vi "Update Main _ Avg Sweeps.vi"() -> ()   [LabVIEW 2022 SP3]
uses:
  Logo.ctl
  C:/Users/Public/OneDrive/Desktop/PMT program/SampleCodeLabView/Kinesis_with_LabVIEW_Examples_LV12 - v3/Thorlabs.MotionControl.Controls.dll
  Kinesis_with_LabVIEW_Examples_LV12 - v3/Thorlabs.MotionControl.Controls.dll
  <vilib>/Utility/file.llb/Write Delimited Spreadsheet (string).vi
  <vilib>/Utility/file.llb/Write Delimited Spreadsheet (I64).vi
  <vilib>/Utility/file.llb/Write Delimited Spreadsheet (DBL).vi
  C:/Users/Public/OneDrive/Desktop/PMT program/SampleCodeLabView/Kinesis_with_LabVIEW_Examples_LV12 - v3/ThorLabs.MotionControl.KCube.DCServoCLI.dll
  Kinesis_with_LabVIEW_Examples_LV12 - v3/ThorLabs.MotionControl.KCube.DCServoCLI.dll
  <vilib>/Analysis/NI_AALBase.lvlib
panel:
  out "RSD":i32=5 caption="Repeat Sweep Data"
  in  "Tab Control":enum32{"Page 1", "Page 2", "Page 3"}(tab)
  out "Sweep Graph":u32[](graph)
  out "Cycled Mean Graph":u32[](graph)
  out "Multiplot":waveform(dbl)[](graph)
  in  "RS":i32=5 caption="Repeat Cycle"
  out "SIND":i32 caption="Total No. of Sweep Iterations"
  out "SIN":i32 caption="Current Sweep Iteration"
  out "ESD":i32=1 caption="Steps\nAdded/Removed"
  in  "ES":i32=1 caption="Add /Remove \nSteps"
  out "SM":i32 caption="Sweep\nMean"
  out "SN":i32 caption="Current  Read Step"
  out "SND":i32 caption="Total No. of Read Steps"
  in  "Auto-Sweep":bool
  in  "P8":bool
  out "PC":i32 caption="Current \nPosition"
  out "WTD":i32=2500 caption="Wait Time (ms)\nRead Data"
  out "EPD":i32=180 caption="End Position\nRead Data"
  out "SPD":i32 caption="Start Position\nRead Data"
  out "SSD":i32=10 caption="Step Size\nRead Data"
  in  "SP":i32 caption="Start Position (degrees)\n Set Data"
  in  "WT":i32=2500 caption="Wait Time (ms)\n Set Data"
  in  "EP":i32=180 caption="End Position (degrees)\n Set Data"
  in  "P7":bool
  in  "SS":i32=10 caption="Step Size (degrees)\nSet Data"
  in  "Motor Controller\nSerialNumber":string="27260805"
  in  "KCubeDCServoControl":refnum<k24>(container)
  in  "Export":bool
  out "DB":u32[](array[numeric])
  out "OVL":bool caption="LED ON : Over Rang Data"
  out "OLD":i32
  out "GN":i32 caption="Gate Number"
  in  "Correction":bool=TRUE
  in  "Logo":T1
  out "Graph":u32[](graph)
  in  "Stop":bool
  in  "Start":bool
  in  "P6":bool
  out "RND":i32=50 caption="Read Number\nRead Data"
  in  "P5":bool
  in  "RN":i32=50 caption="Read Number\nSet Data"
  out "PowerD":i32 caption="Power\nRead Data"
  out "ITD":i32=40 caption="Internal Time\nRead Data"
  in  "P4":bool
  in  "P3":bool
  in  "IT":i32=40 caption="Internal Time\nSet Data"
  in  "P2":bool
  out "Handle Number":i32
  in  "P1":bool caption="Switch\nPower OFF/Power ON"
  in  "EXIT":bool
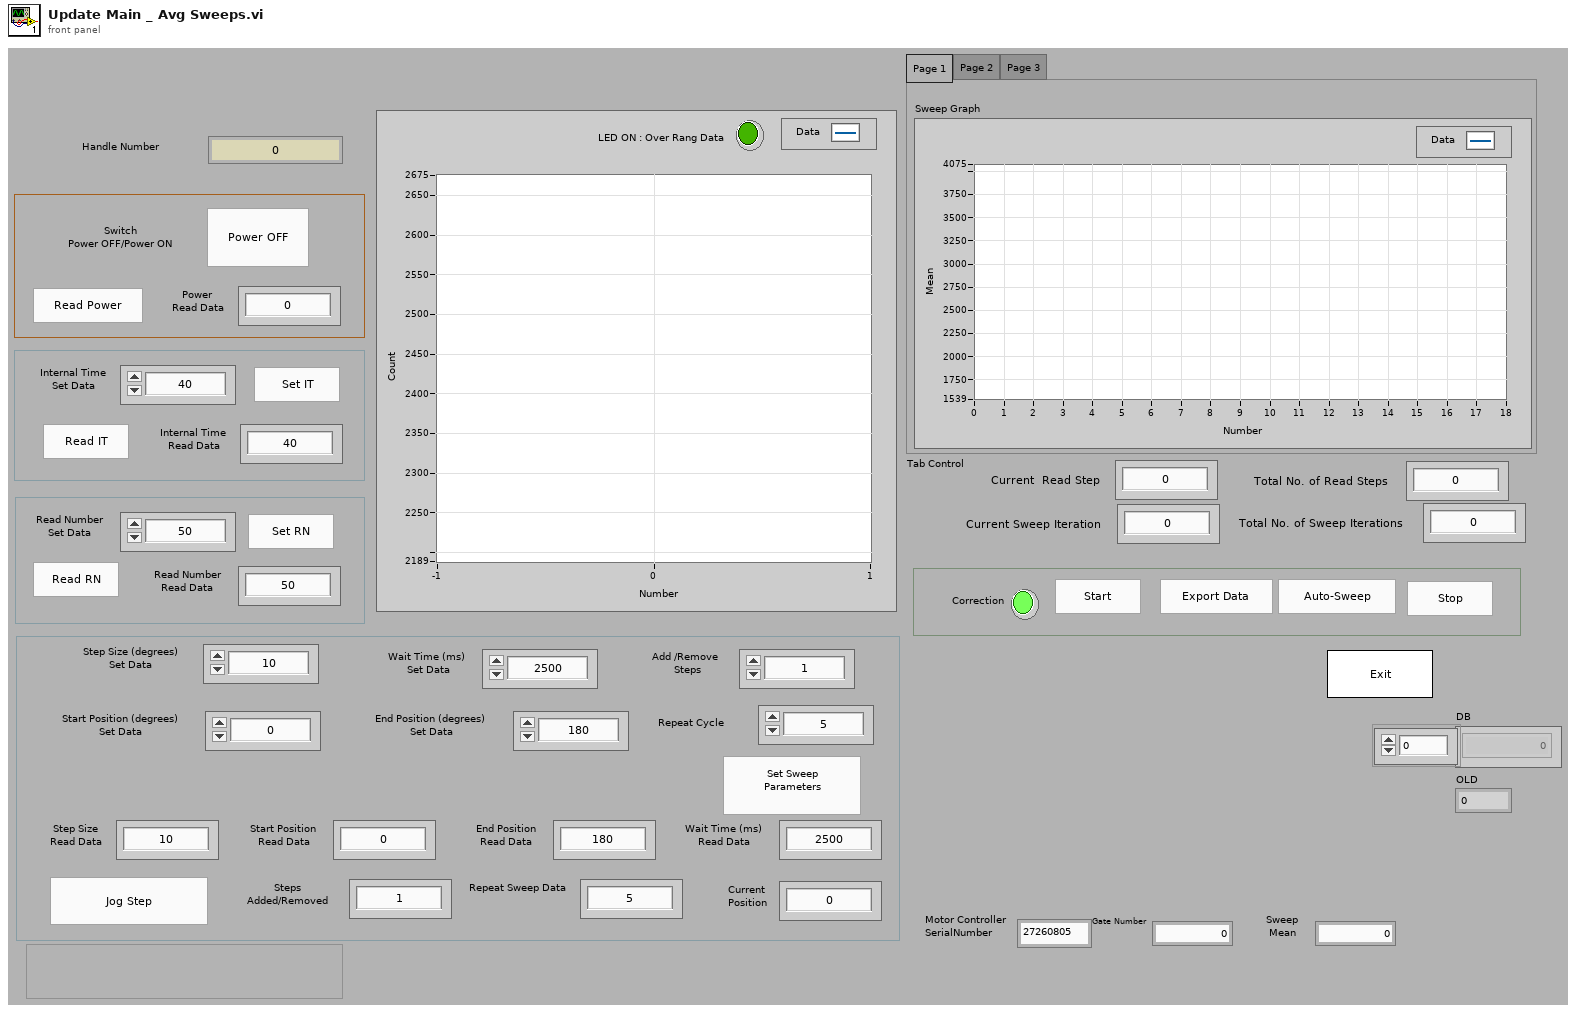
[diagram p1: front panel]
types:
  T1 = typedef "Logo.ctl" = bool
  T2 = enum8{"Enabled", "Disabled", "Disabled and Grayed Out"}
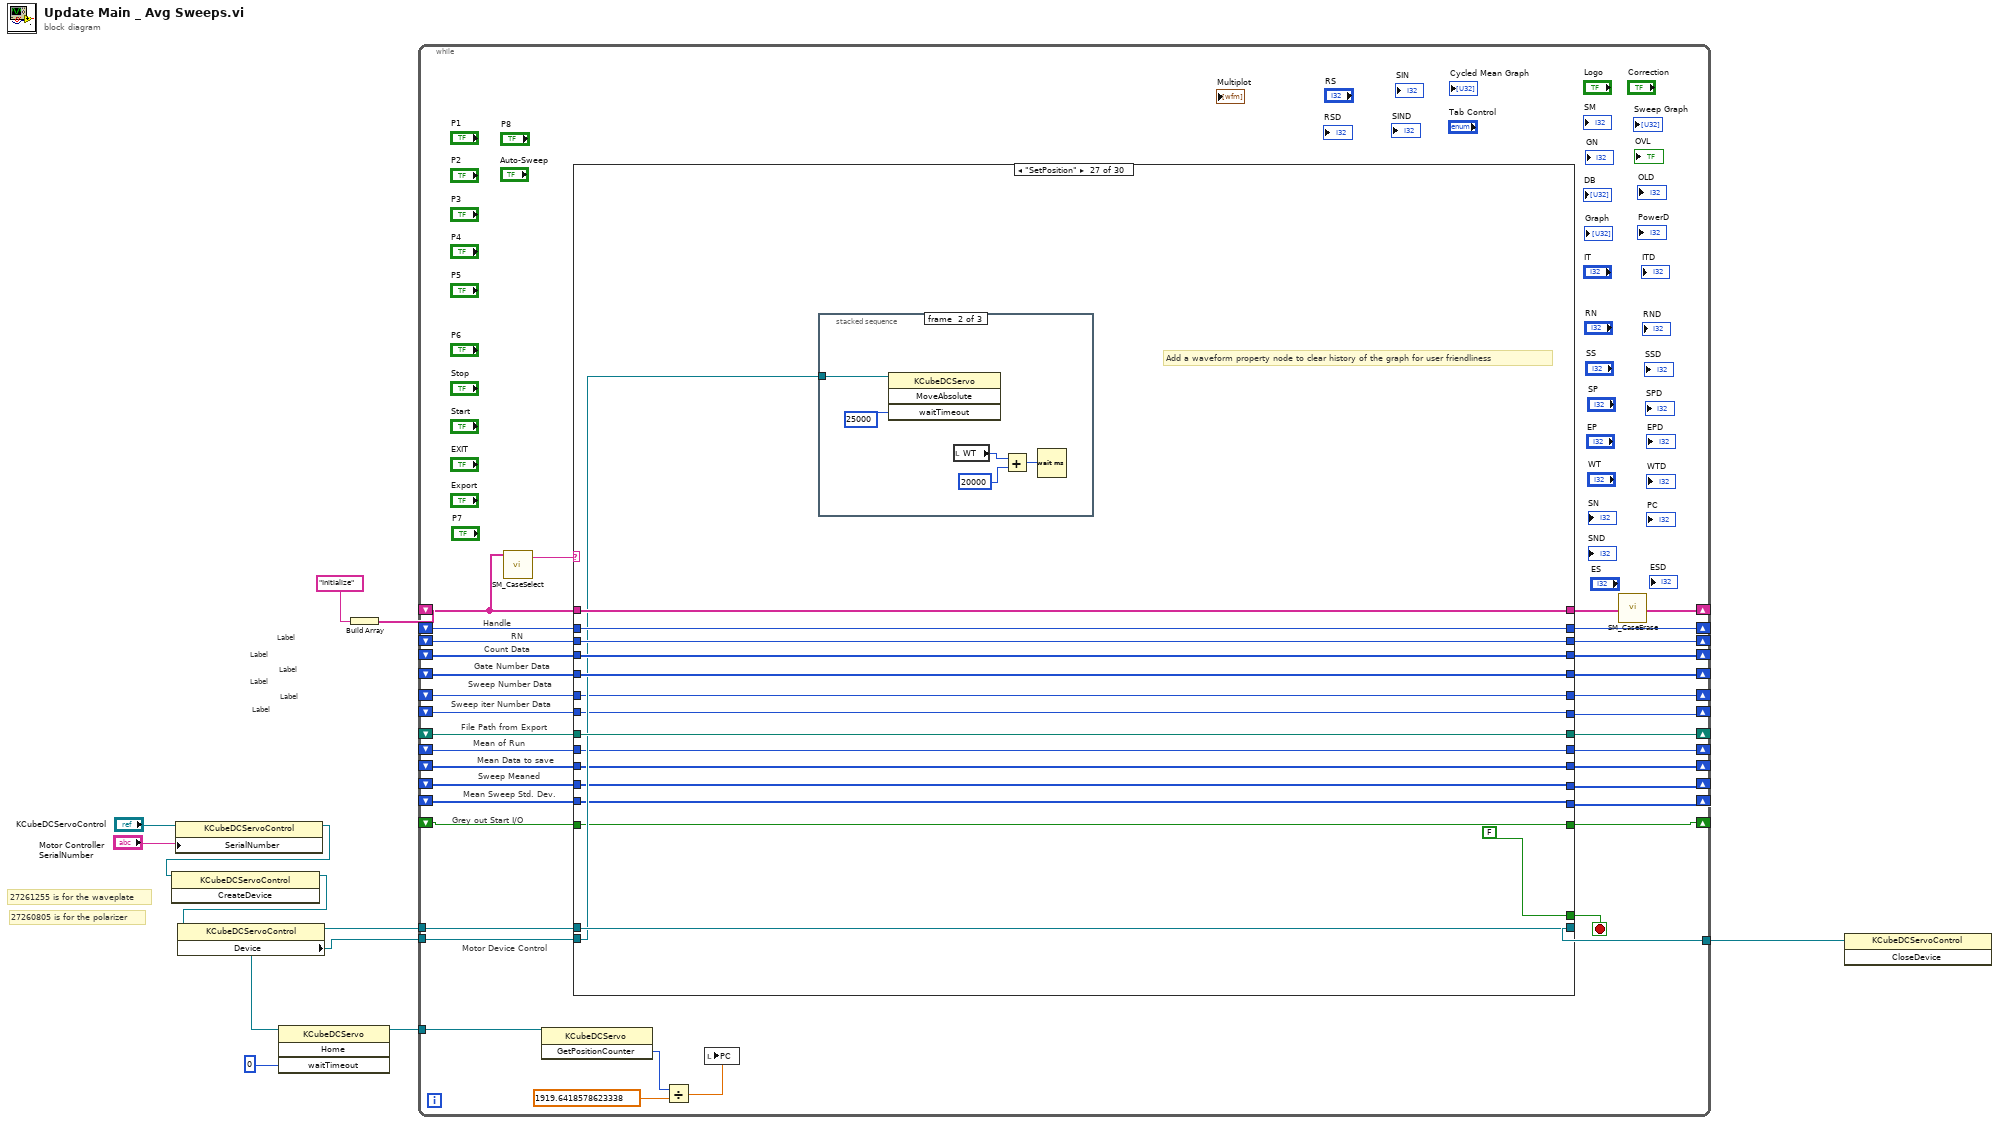
[diagram p0: block diagram]
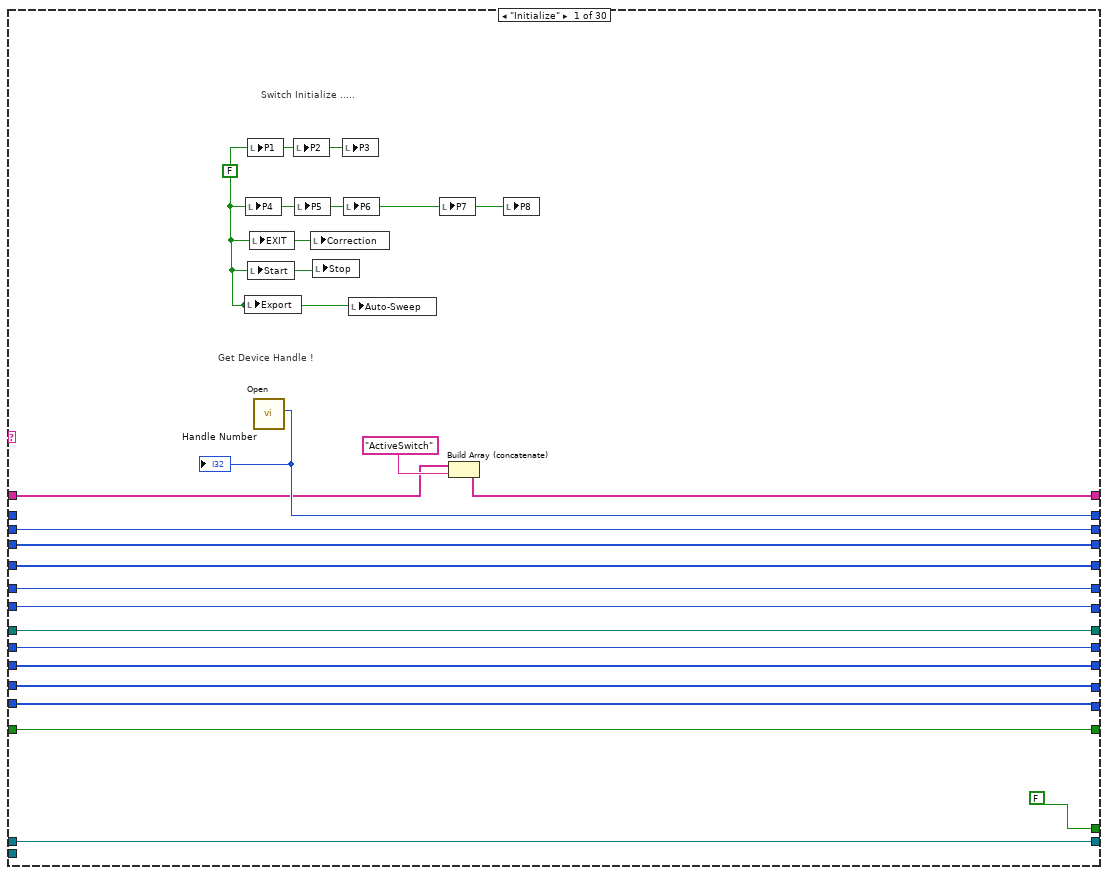
[diagram p2: hidden frame]
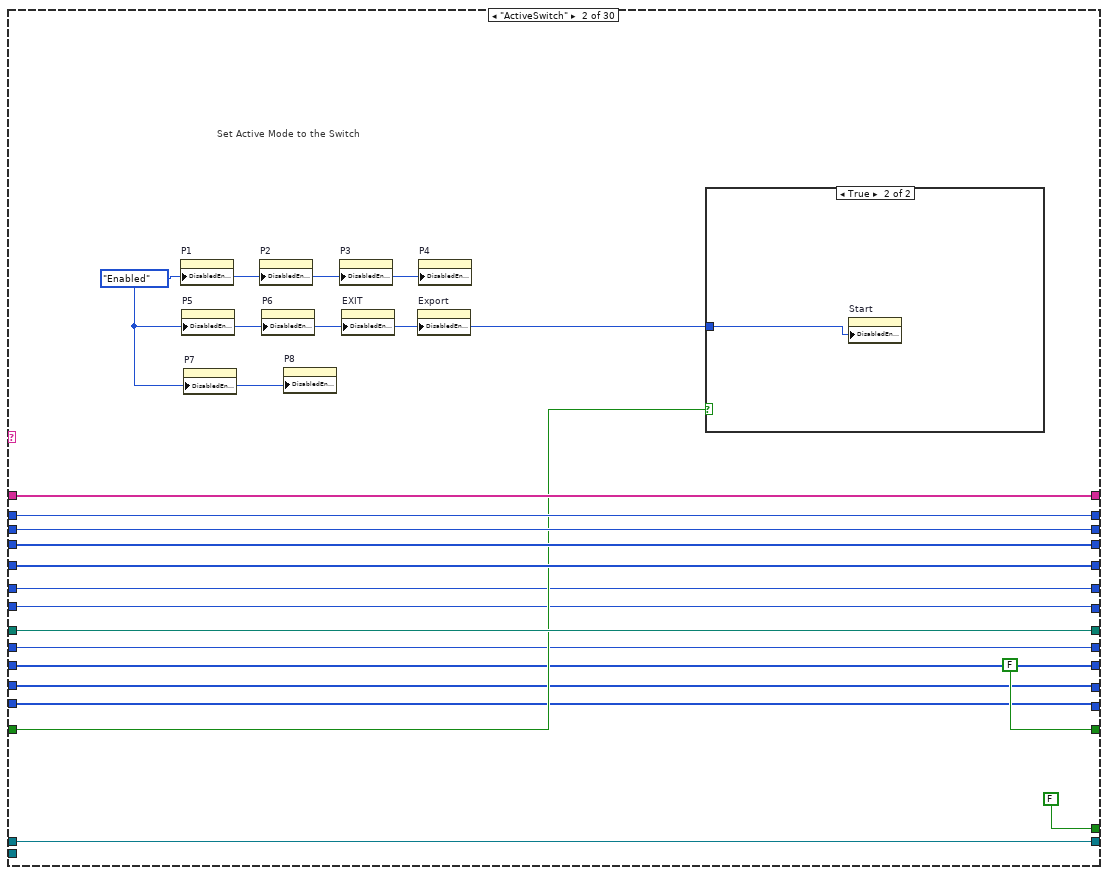
[diagram p3: hidden frame]
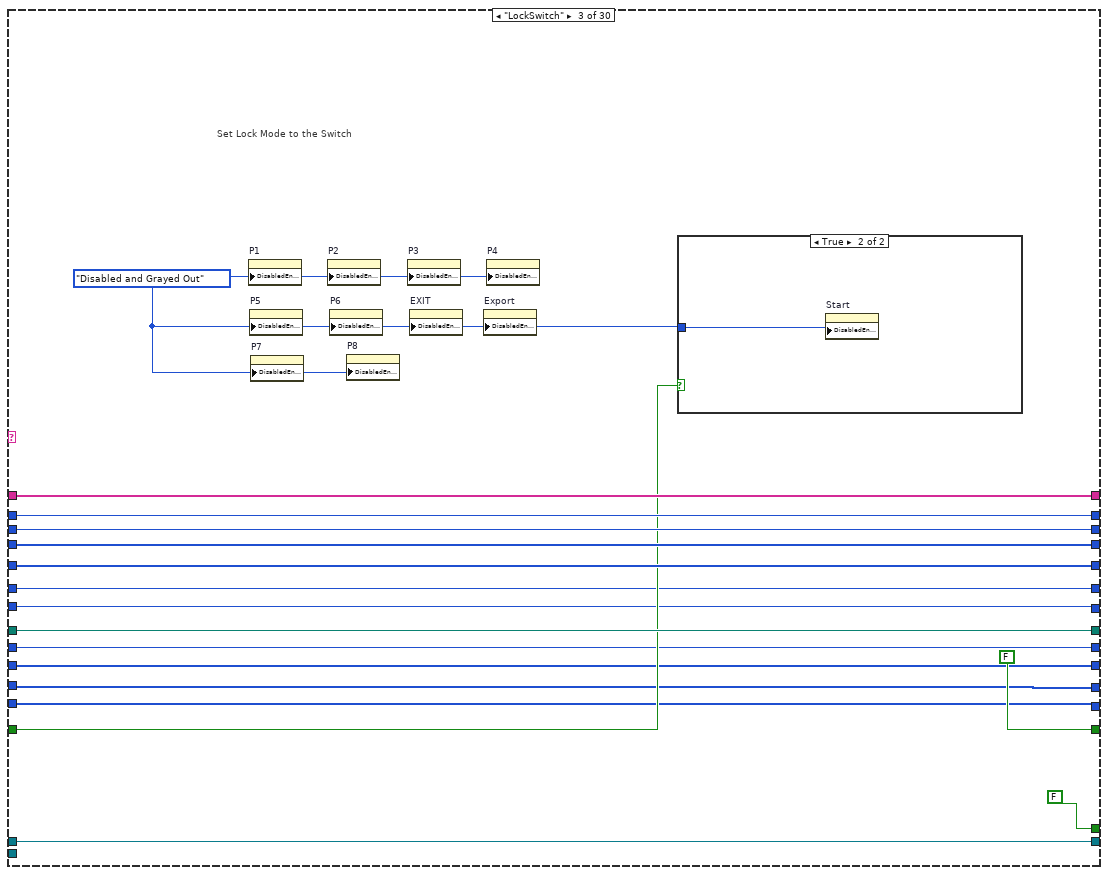
[diagram p5: hidden frame]
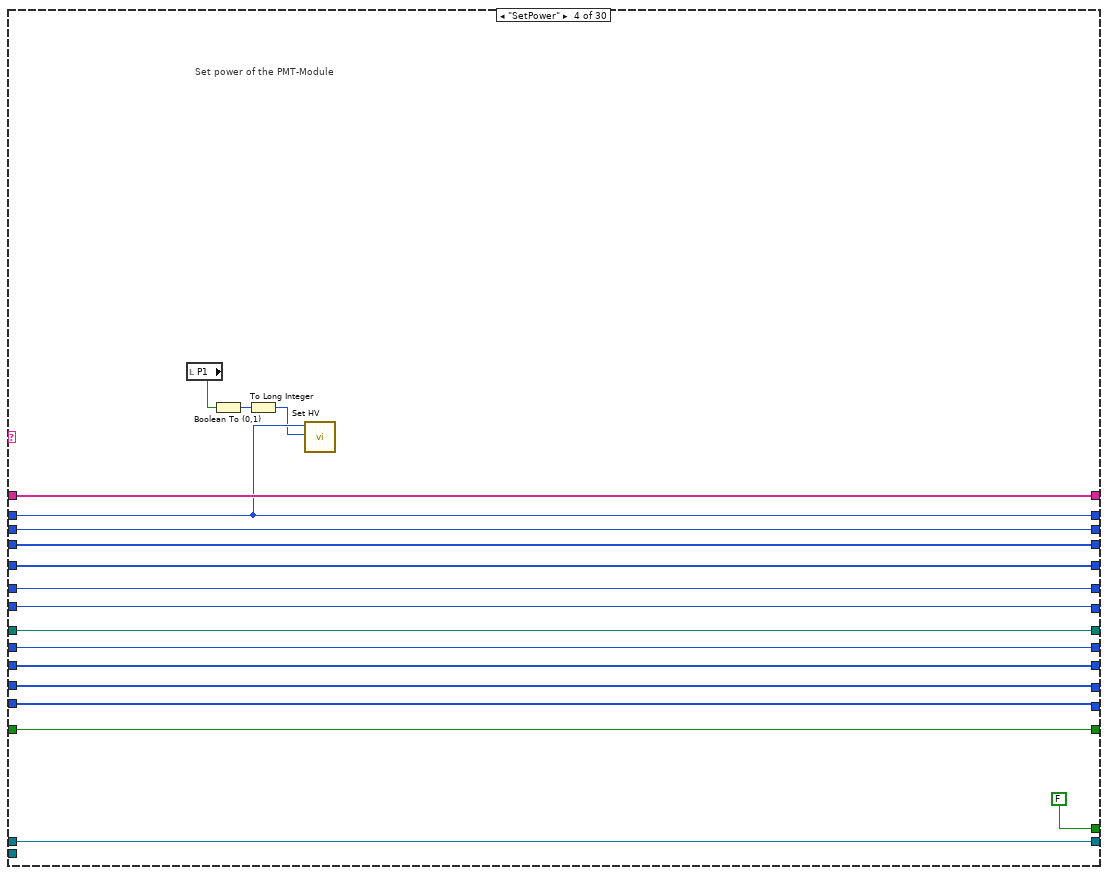
[diagram p7: hidden frame]
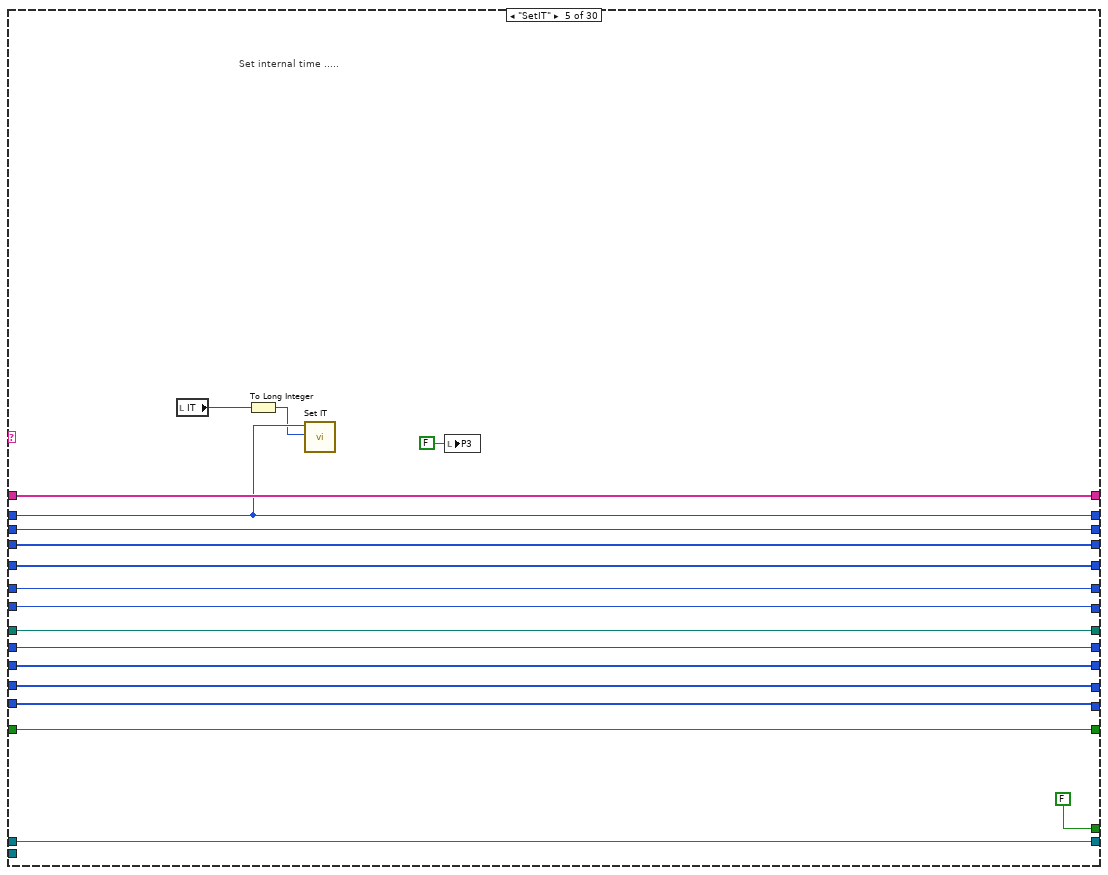
[diagram p8: hidden frame]
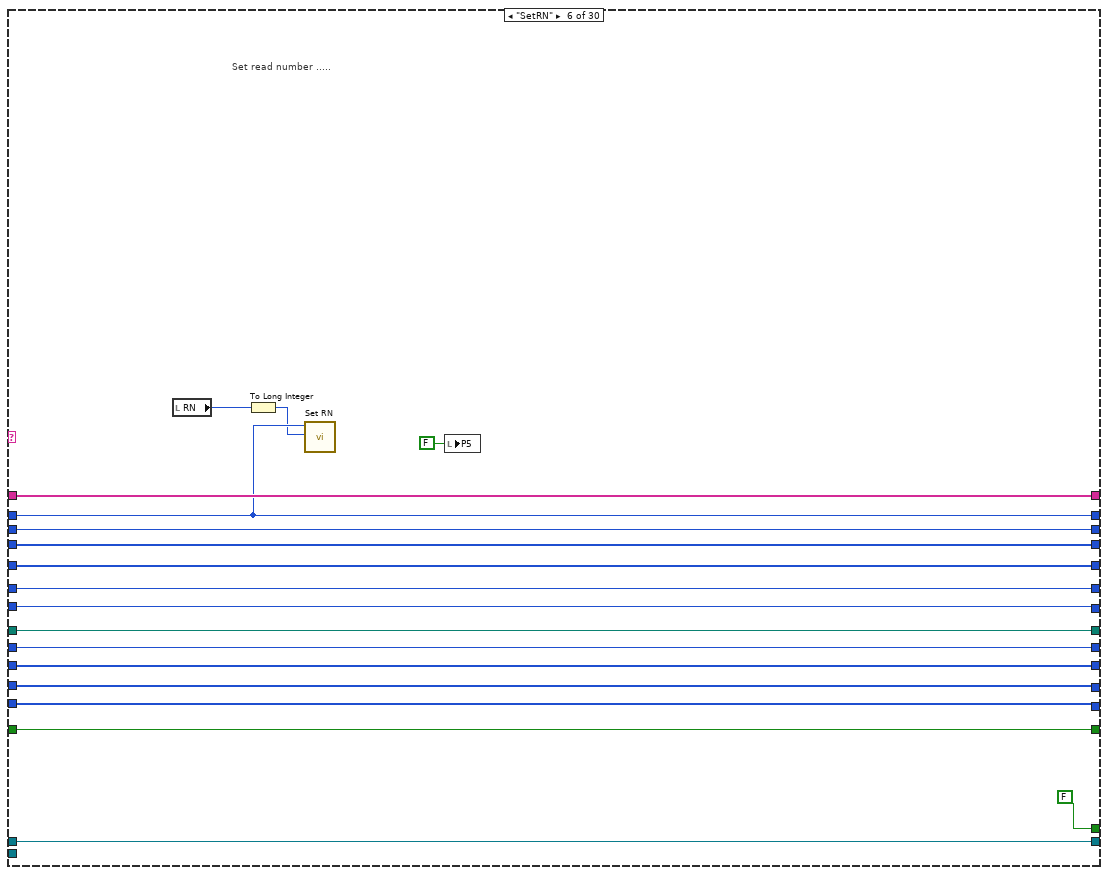
[diagram p9: hidden frame]
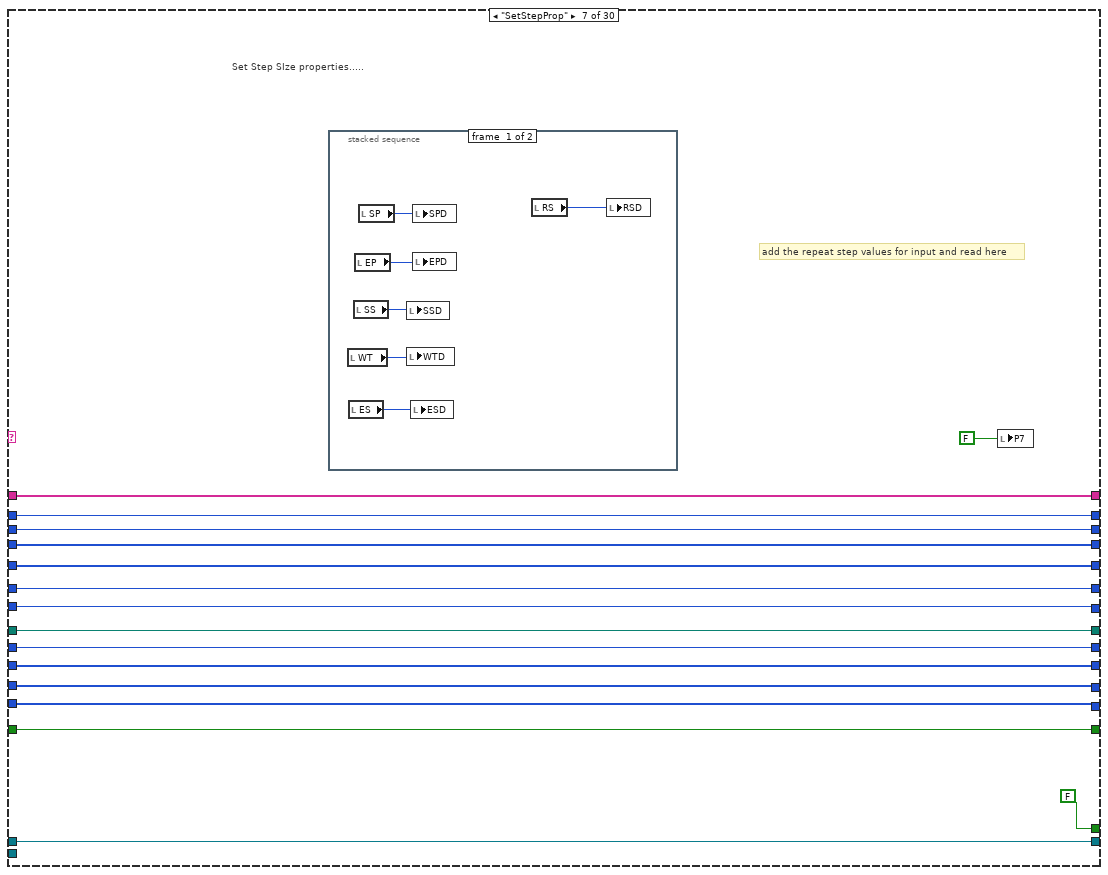
[diagram p10: hidden frame]
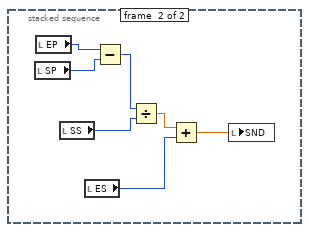
[diagram p11: hidden frame]
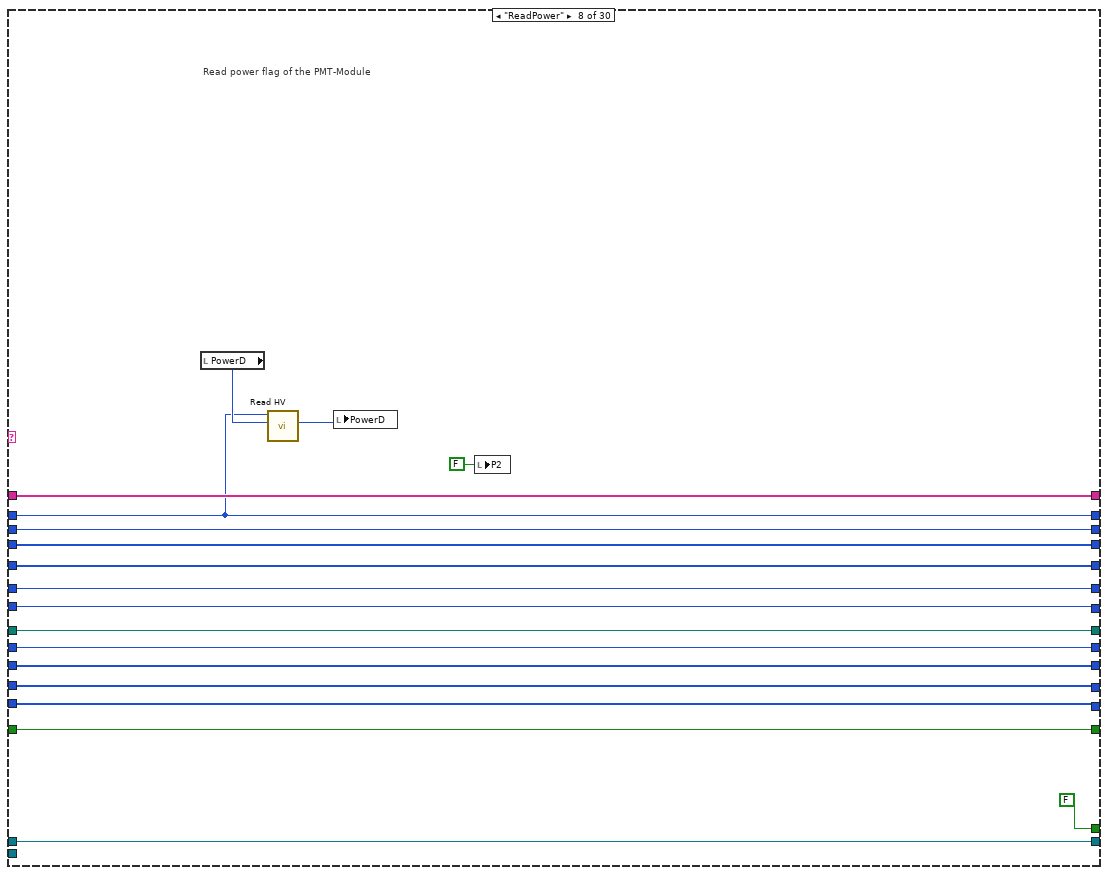
[diagram p12: hidden frame]
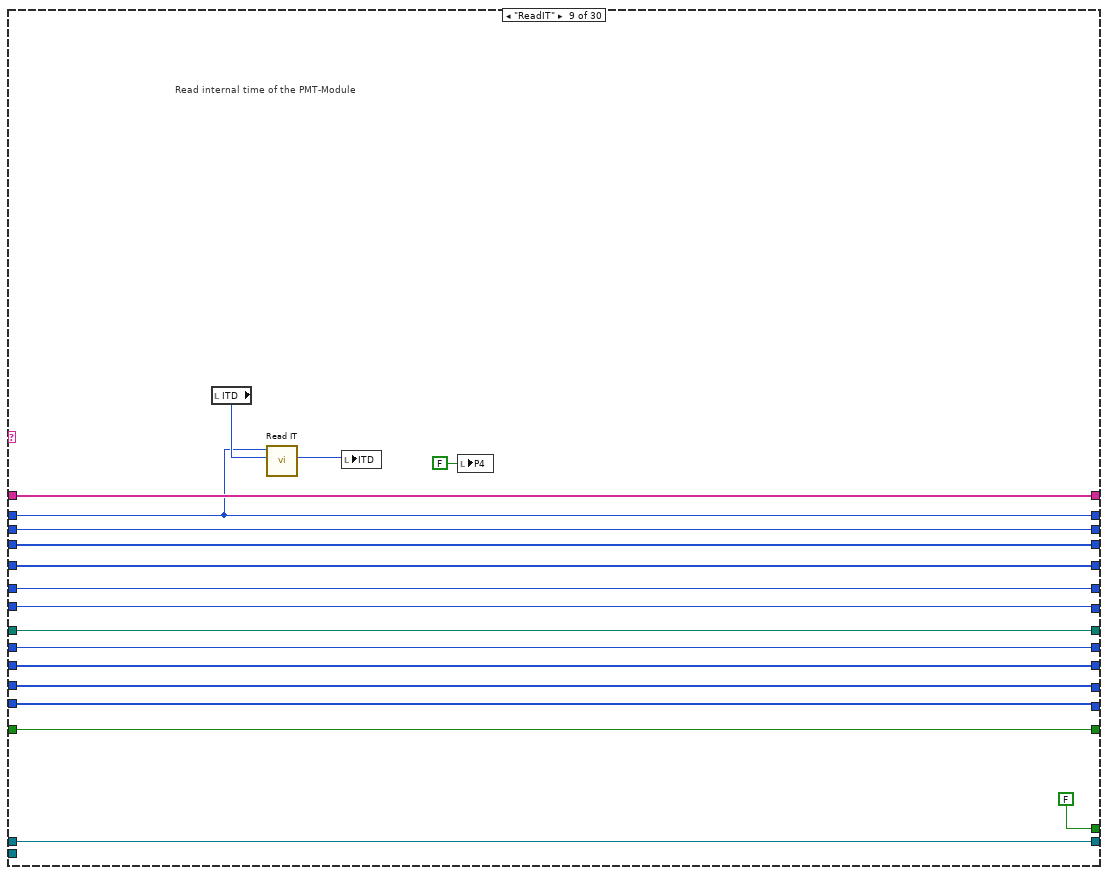
[diagram p13: hidden frame]
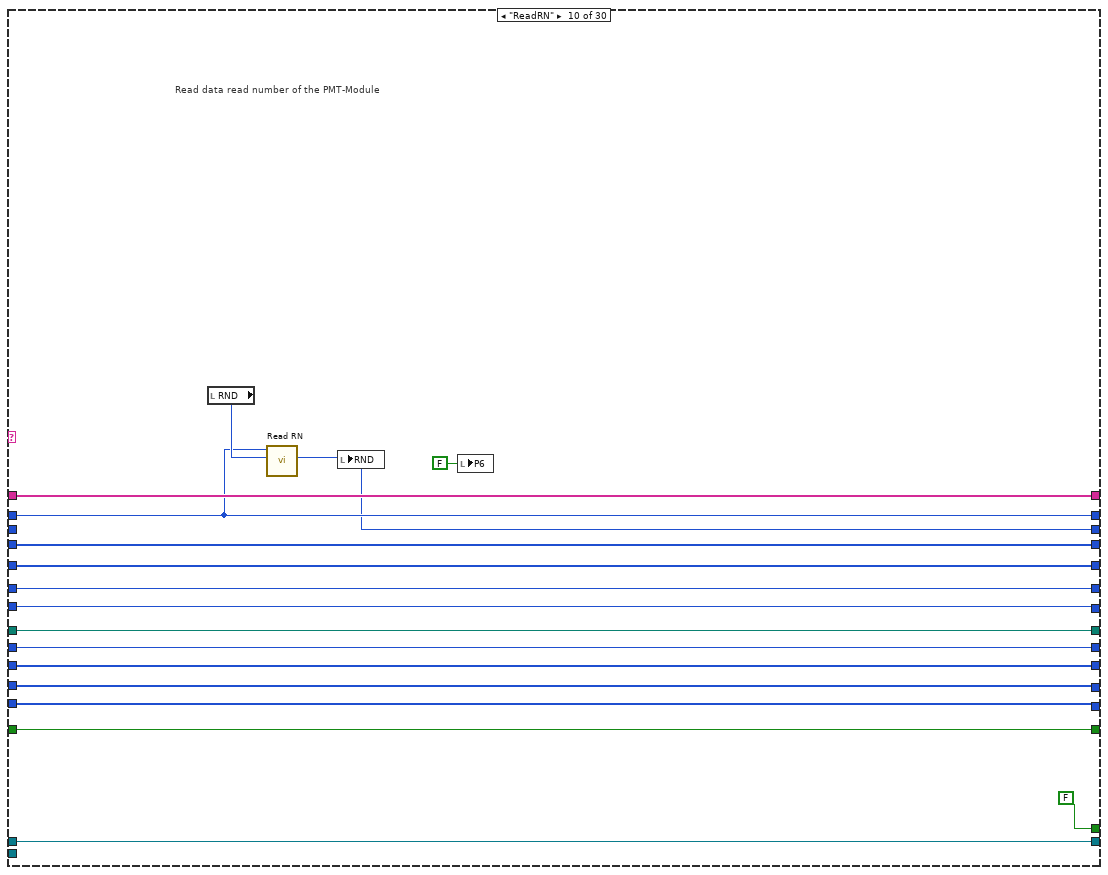
[diagram p14: hidden frame]
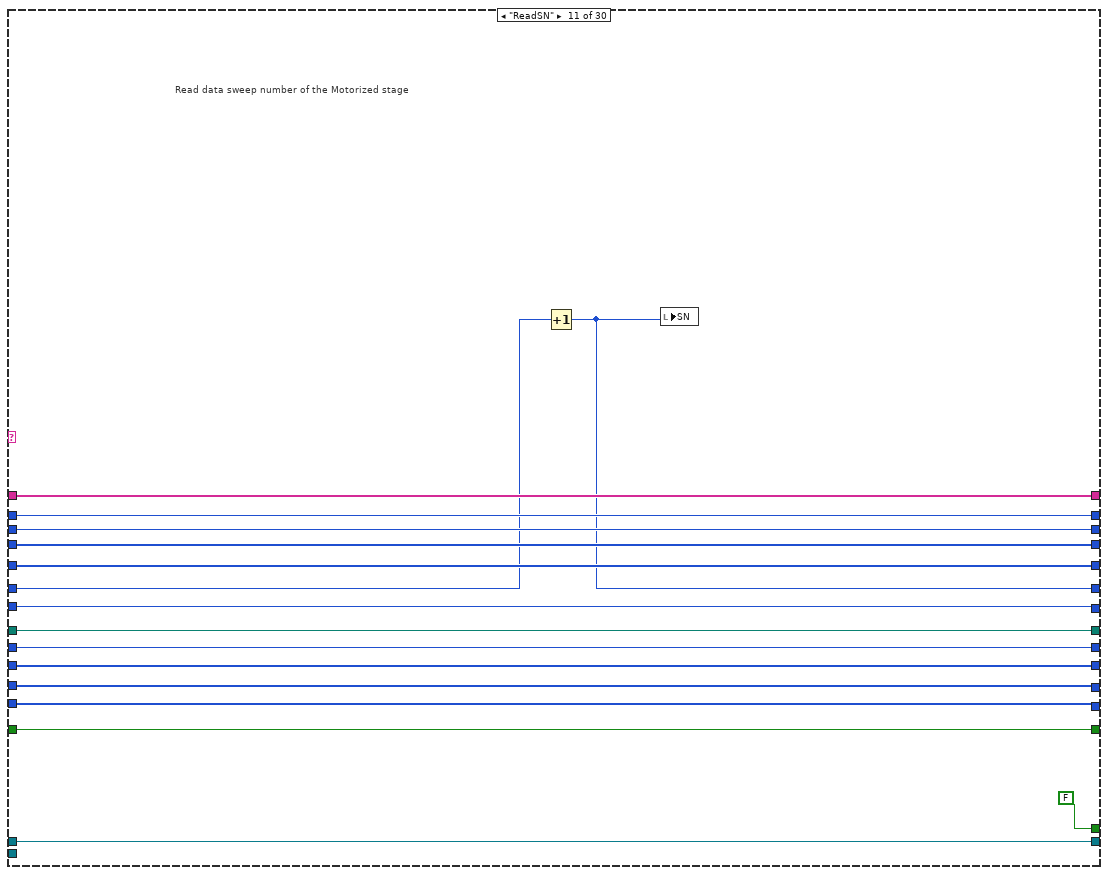
[diagram p15: hidden frame]
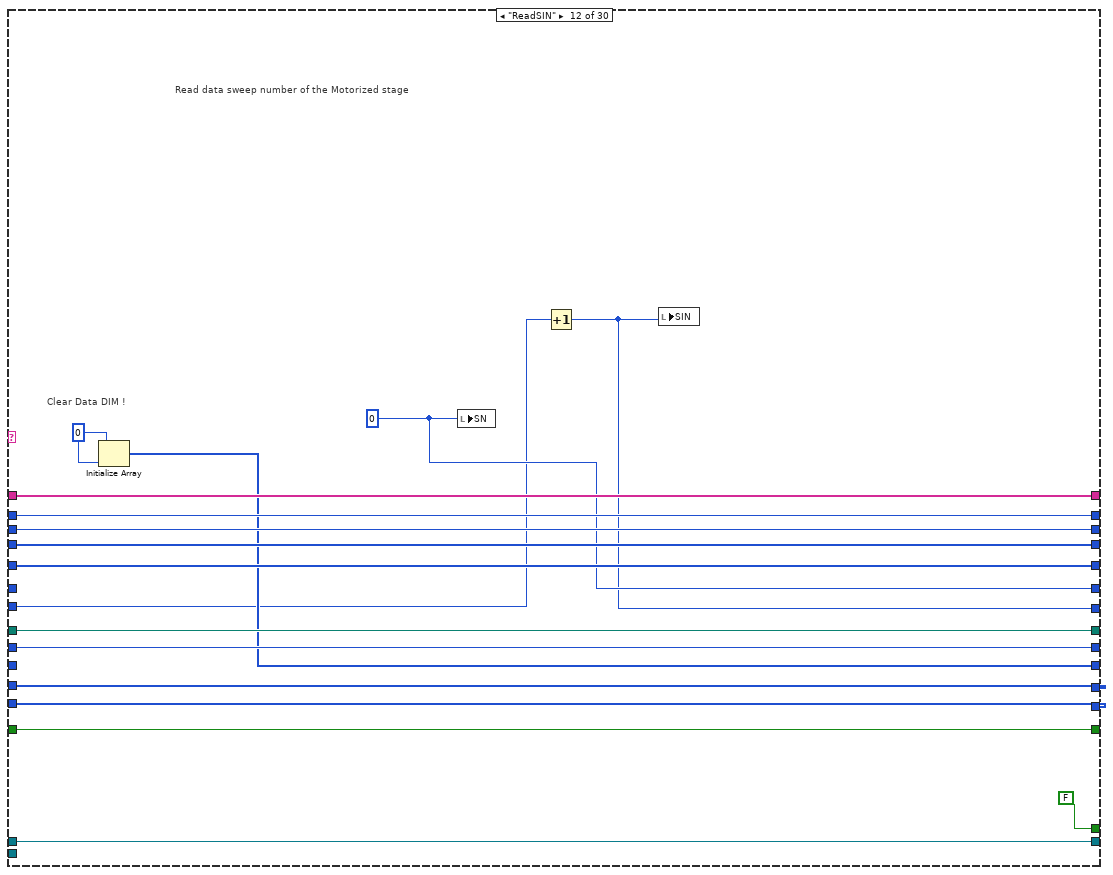
[diagram p16: hidden frame]
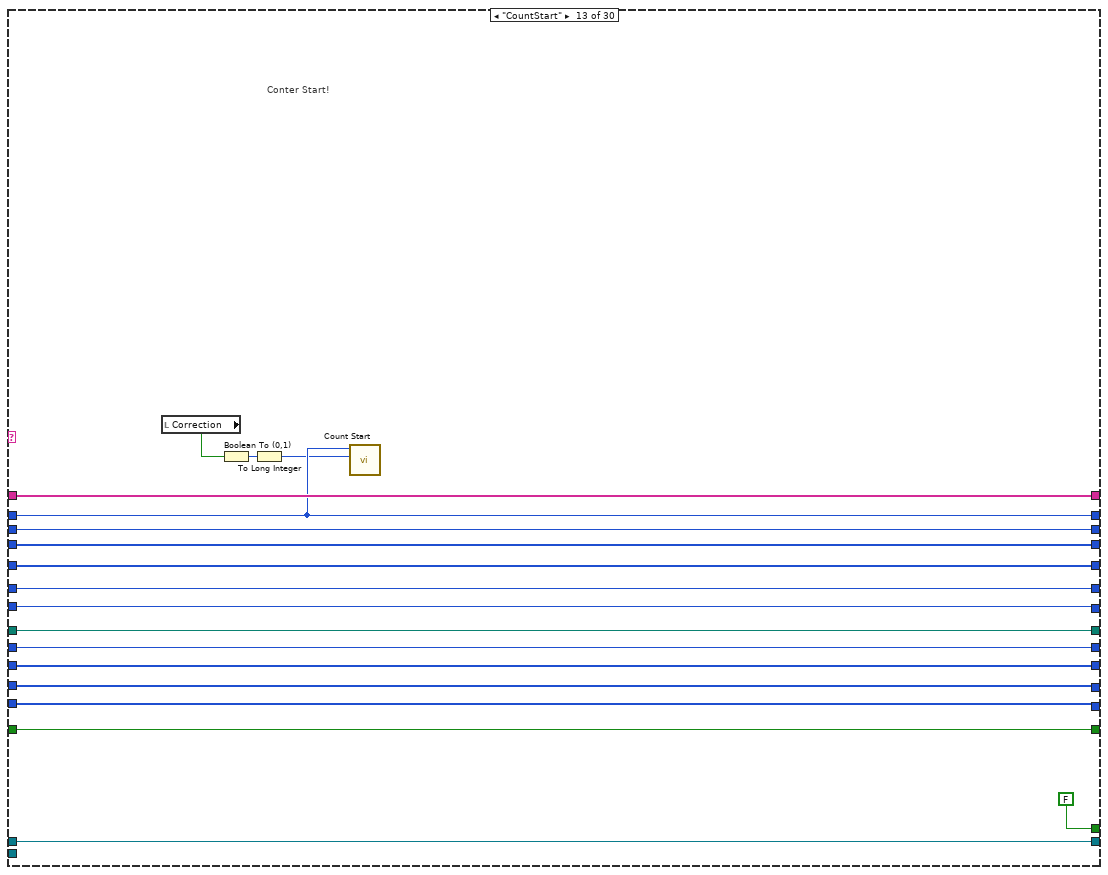
[diagram p17: hidden frame]
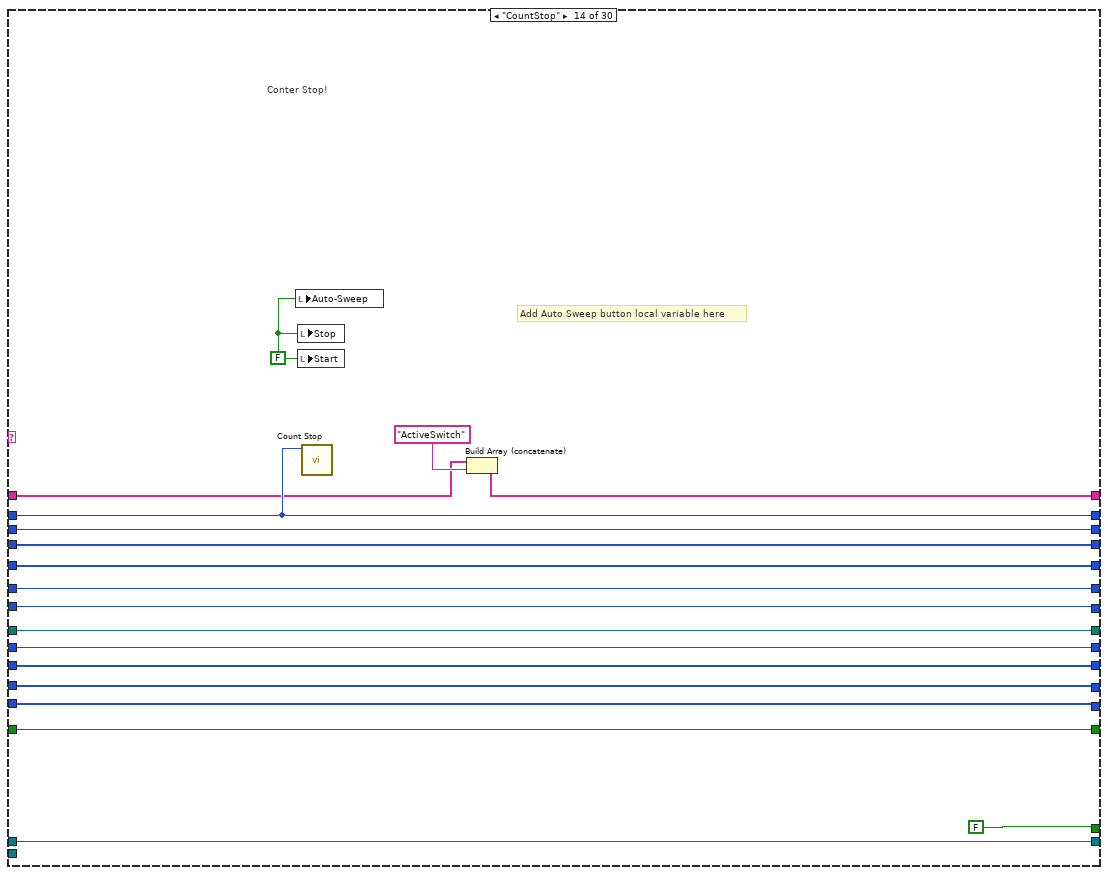
[diagram p18: hidden frame]
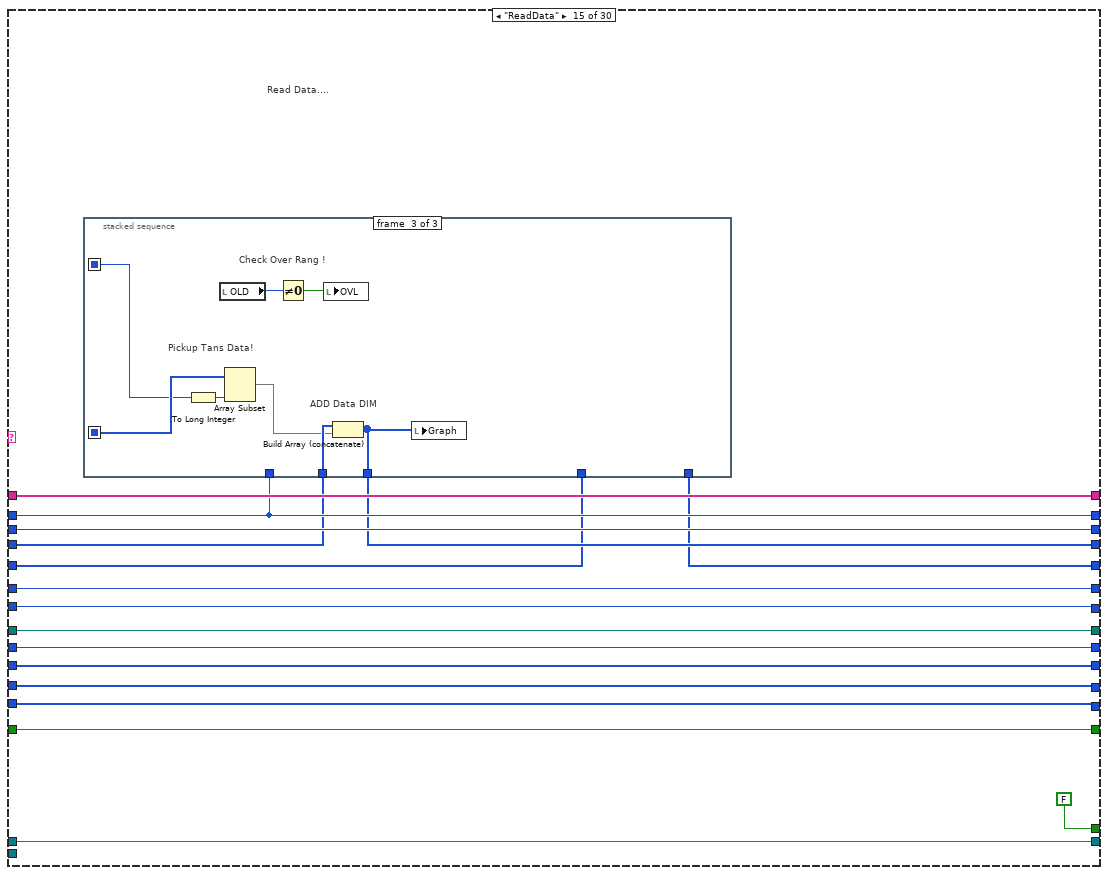
[diagram p19: hidden frame]
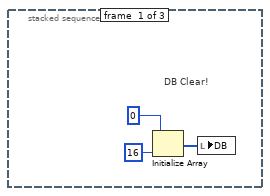
[diagram p20: hidden frame]
diagram:
  # "27260805 is for the polarizer"
  # "27261255 is for the waveplate"
  # "Label"
  # "Label"
  # "Label"
  # "Label"
  # "Label"
  # "Label"
  n1 = property class="KCubeDCServoControl"(reference="KCubeDCServoControl", "SerialNumber"="Motor Controller\nSerialNumber") -> (reference out=w8:refnum<k24>)  [unwired: 1 in, 1 out]
  n2 = invoke class="KCubeDCServoControl" method="CreateDevice"(reference=w8) -> (reference out=w1:refnum<k24>)  [unwired: 2 in, 2 out]
  n3 = property class="KCubeDCServoControl"(reference=w1) -> (reference out=w5:refnum<k24>, "Device"=w3:refnum<k24>)  [unwired: 1 in, 1 out]
  n4 = invoke class="KCubeDCServo" method="Home"(reference=w3, "waitTimeout"=0) -> (reference out=w2:refnum<k24>)  [unwired: 2 in, 3 out]
  n5 = Build Array("Initialize") -> (w10:string[])
  n6 = while {
    shift-right: [w40] -> _
    shift-left: _ -> [w41]
    shift-right: [w42] -> _
    shift-left: _ -> [w43]
    shift-right: [w44] -> _
    shift-left: _ -> [w45]
    shift-right: [w37] -> _
    shift-left: w10 -> [w46]
    tunnel: w5 -> [w34]
    tunnel: [w33] -> w6
    shift-right: [w36] -> _
    shift-left: _ -> [w35]
    tunnel: w3 -> [w32]
    shift-right: [w31] -> _
    shift-left: _ -> [w30]
    shift-right: [w29] -> _
    shift-left: _ -> [w28]
    tunnel: w2 -> [w27]
    shift-right: [w25] -> _
    shift-left: _ -> [w26]
    shift-right: [w24] -> _
    shift-left: _ -> [w23]
    shift-right: [w22] -> _
    shift-left: _ -> [w21]
    shift-right: [w17] -> _
    shift-left: _ -> [w16]
    shift-right: [w15] -> _
    shift-left: _ -> [w14]
    shift-right: [w13] -> _
    shift-left: _ -> [w12]
    stop <- w39 stop-if-true
    # "Sweep iter Number Data"
    # "Mean Sweep Std. Dev."
    # "Sweep Meaned"
    # "Mean Data to save"
    # "Mean of Run"
    # "Sweep Number Data"
    # "Grey out Start I/O"
    # "Motor Device Control"
    # "File Path from Export"
    # "Gate Number Data"
    # "Count Data"
    # "RN"
    # "Handle"
    n7 = call "SM_CaseSelect.vi"("Input"=w46) -> ("Case"=w47:string)  [unwired: 10 out]
    n8 = invoke class="KCubeDCServo" method="GetPositionCounter"(reference=w27) -> ("GetPositionCounter"=w19:i32)  [unwired: 2 in, 2 out]
    n9 = case shown="\"SetPosition\"" w47 {
      selector: w47 -> [_ _ _ _ _ _ _ _ _ _ _ _ _ _ _ _ _ _ _ _ _ _ _ _ _ _ _ _ w873 _]
      tunnel: w46 -> [w60 w82 w100 w119 w137 w155 w171 w202 w220 w237 w253 w270 w288 w301 w323 w361 w398 w408 w451 w484 w575 w623 w670 w714 w722 w761 w787 w814 w882 w897]
      tunnel: [w59 w82 w100 w119 w137 w155 w171 w202 w220 w237 w253 w270 w288 w300 w323 w361 w397 w407 w452 w485 w575 w623 w670 w714 w721 w761 w787 w811 w882 w897] -> w38
      tunnel: w45 -> [_ w78 w96 w115 w133 w151 w167 w197 w215 w233 w250 w267 w284 w303 w320 w358 w399 w419 w454 w486 w574 w622 w669 w713 w734 w760 w786 w817 w881 w893]
      tunnel: [w62 w78 w96 w115 w133 w151 w167 w197 w215 w233 w250 w267 w284 w303 w320 w358 w399 w419 w454 w486 w574 w622 w669 w713 w734 w760 w786 w817 w881 w893] -> w44
      tunnel: w43 -> [w65 w81 w99 w118 w136 w154 w170 w201 w219 _ w243 w261 w287 w306 w322 w360 w401 w421 w449 w482 w573 w621 w668 w712 w733 w759 w785 w816 w880 w896]
      tunnel: [w65 w81 w99 w118 w136 w154 w170 w201 w219 w231 w243 w261 w287 w306 w322 w360 w401 w421 w449 w482 w573 w621 w668 w712 w733 w759 w785 w816 w880 w896] -> w42
      tunnel: w41 -> [w64 w80 w98 w117 w135 w153 w169 w200 w218 w236 w252 w269 w286 w305 w319 w353 _ _ w445 w480 w558 w606 w653 w703 w732 w758 w784 w810 w879 w895]
      tunnel: [w64 w80 w98 w117 w135 w153 w169 w200 w218 w236 w252 w269 w286 w305 w318 w353 w389 w417 w445 w480 w558 w606 w653 w703 w732 w758 w784 w810 w879 w895] -> w40
      tunnel: [FALSE FALSE FALSE FALSE FALSE FALSE FALSE FALSE FALSE FALSE FALSE FALSE FALSE FALSE FALSE FALSE FALSE FALSE FALSE FALSE FALSE FALSE FALSE FALSE FALSE FALSE FALSE FALSE FALSE TRUE] -> w39
      tunnel: [w58 w77 w95 w111 w129 w147 w166 w194 w212 w230 w249 w266 w280 w299 w317 w352 w389 w417 w444 w479 w553 w601 w648 w698 w731 w757 w783 w809 w872 w892] -> w36
      tunnel: w35 -> [w58 w77 w95 w111 w129 w147 w166 w194 w212 w230 w249 w266 w280 w299 w316 w352 _ _ w444 w479 w553 w601 w648 w698 w731 w757 w783 w809 w872 w892]
      tunnel: w34 -> [w57 w76 w94 w110 w128 w146 w165 w193 w211 w229 w248 w265 w279 w298 w315 w357 w388 w416 w443 w478 w555 w603 w650 w700 w730 w756 w782 w808 w871 w891]
      tunnel: [w57 w76 w94 w110 w128 w146 w165 w193 w211 w229 w248 w265 w279 w298 w315 w357 w388 w416 w443 w478 w555 w603 w650 w700 w730 w756 w782 w808 w871 w891] -> w33
      tunnel: w32 -> [_ _ _ _ _ _ _ _ _ _ _ _ _ _ _ _ _ _ _ _ _ _ _ _ _ w753 w779 _ _ _]
      tunnel: [w56 w75 w93 w109 w127 w145 w163 w192 w210 w228 w247 w264 w278 w297 w314 w356 w387 w415 w442 w477 w546 w597 w644 w693 w723 w754 w780 w807 w870 w890] -> w31
      tunnel: w30 -> [w56 w75 w93 w109 w127 w145 w163 w192 w210 w228 w247 w264 w278 w297 w314 w356 w387 w415 w442 w477 w546 w595 w642 w687 _ w754 w780 w807 w870 w890]
      tunnel: [w55 FALSE FALSE w108 w126 w144 w162 w191 w209 w227 w246 w263 w277 w296 w313 w355 w386 TRUE w441 w476 w548 w596 w643 w697 w728 w752 w778 w806 w869 w889] -> w29
      tunnel: w28 -> [w55 w74 w92 w108 w126 w144 w162 w191 w209 w227 w246 w263 w277 w296 w313 w355 w386 _ w441 _ w548 w596 w643 w697 w728 w752 w778 w806 w869 w889]
      tunnel: w26 -> [w53 w71 w89 w107 w125 w143 w161 w190 w208 w226 w241 _ w276 w295 w312 w354 w385 w413 w440 w475 w547 w591 w641 w696 _ w748 w777 w805 w868 w888]
      tunnel: [w53 w71 w89 w107 w125 w143 w161 w190 w208 w226 w242 w256 w276 w295 w312 w354 w385 w413 w440 w475 w547 w591 w641 w696 w720 w748 w777 w805 w868 w888] -> w25
      tunnel: [w52 w70 w88 w106 w124 w142 w160 w189 w207 w225 w245 w262 w275 w294 w311 w351 w384 w412 w439 w474 w545 w581 w635 w695 w727 w750 w776 w804 w867 w887] -> w24
      tunnel: w23 -> [w52 w70 w88 w106 w124 w142 w160 w189 w207 w225 w245 w262 w275 w294 w311 w351 w384 w412 w439 w474 w545 _ _ w695 w727 w750 w776 w804 w867 w887]
      tunnel: [w51 w69 w87 w105 w123 w141 w159 w188 w206 w224 w244 w257 w274 w293 w310 w350 w383 w411 w438 w473 w544 w586 w636 w694 w726 w749 w775 w803 w866 w886] -> w22
      tunnel: w21 -> [w51 w69 w87 w105 w123 w141 w159 w188 w206 w224 w244 _ w274 w293 w310 w349 w383 w411 w438 w473 w544 w586 w636 w694 w726 w749 w775 w803 w866 w886]
      tunnel: [w50 w68 w86 w104 w122 w140 w158 w187 w205 w223 w240 w260 w273 w291 w309 w348 w382 w404 w437 w472 w543 w585 w639 w691 w725 w747 w774 w802 w865 w885] -> w17
      tunnel: w16 -> [w50 w68 w86 w104 w122 w140 w158 w187 w205 w223 w240 w260 w273 w291 w309 w348 w382 w404 w437 w472 w543 w585 _ w691 w725 w747 w774 w802 w865 w885]
      tunnel: [w49 w67 w85 w103 w121 w139 w157 w186 w204 w222 w239 w259 w272 w290 w308 w347 w381 w403 w436 w471 w542 w584 w638 w692 w724 w746 w773 w801 w864 w884] -> w15
      tunnel: w14 -> [w49 w67 w85 w103 w121 w139 w157 w186 w204 w222 w239 w259 w272 w290 w308 w347 w381 w403 w436 w471 w542 w584 _ w692 w724 w746 w773 w801 w864 w884]
      tunnel: [w48 w66 w84 w102 w120 w138 w156 w185 w203 w221 w238 w255 w271 w289 w307 w346 w380 w402 w435 w467 w541 w583 w637 w685 w720 w745 w772 w800 w863 w883] -> w13
      tunnel: w12 -> [w48 w66 w84 w102 w120 w138 w156 w185 w203 w221 w238 w254 w271 w289 w307 w346 w380 w402 w435 w467 w541 w583 w637 w685 _ w745 w772 w800 w863 w883]
      frame "Initialize" {
        w54 = FALSE ("P1")
        # "Get Device Handle !"
        # "Switch Initialize ....."
        n10 = local write "Export"(w54) -> ()
        n11 = local write "P4"(w54) -> ()
        n12 = local write "P1"(w54) -> ()
        n13 = local write "Start"(w54) -> ()
        n14 = local write "EXIT"(w54) -> ()
        n15 = call "Open.vi"() -> ("Handle Number"=w62:i32)  [unwired: 10 in, 1 out]
        "Handle Number" <- w62
        n16 = local write "P2"(w54) -> ()
        n17 = local write "P5"(w54) -> ()
        n18 = local write "Correction"(w54) -> ()
        n19 = local write "Stop"(w54) -> ()
        n20 = local write "P3"(w54) -> ()
        n21 = local write "P6"(w54) -> ()
        n22 = local write "Auto-Sweep"(w54) -> ()
        n23 = local write "P7"(w54) -> ()
        n24 = Build Array (concatenate)(w60, "ActiveSwitch") -> (w59:string[])
        n25 = local write "P8"(w54) -> ()
      }
      frame "ActiveSwitch" {
        w72 = T2."Enabled" ("無効")
        # "Set Active Mode to the Switch"
        n26 = property on="P1" class="Bool (strict)"("DisabledEnum"=w72) -> ()  [unwired: 2 in, 2 out]
        n27 = property on="P5" class="Bool (strict)"("DisabledEnum"=w72) -> ()  [unwired: 2 in, 2 out]
        n28 = property on="P7" class="Bool (strict)"("DisabledEnum"=w72) -> ()  [unwired: 2 in, 2 out]
        n29 = property on="P2" class="Bool (strict)"("DisabledEnum"=w72) -> ()  [unwired: 2 in, 2 out]
        n30 = property on="P6" class="Bool (strict)"("DisabledEnum"=w72) -> ()  [unwired: 2 in, 2 out]
        n31 = property on="P8" class="Bool (strict)"("DisabledEnum"=w72) -> ()  [unwired: 2 in, 2 out]
        n32 = property on="P3" class="Bool (strict)"("DisabledEnum"=w72) -> ()  [unwired: 2 in, 2 out]
        n33 = property on="EXIT" class="Bool (strict)"("DisabledEnum"=w72) -> ()  [unwired: 2 in, 2 out]
        n34 = property on="Export" class="Bool (strict)"("DisabledEnum"=w72) -> ()  [unwired: 2 in, 2 out]
        n35 = property on="P4" class="Bool (strict)"("DisabledEnum"=w72) -> ()  [unwired: 2 in, 2 out]
        n36 = case shown="True" w74 {
          tunnel: w72 -> [_ w83]
          frame False {
          }
          frame True {
            n37 = property on="Start" class="Bool (strict)"("DisabledEnum"=w83) -> ()  [unwired: 2 in, 2 out]
          }
        }
      }
      frame "LockSwitch" {
        w90 = T2."Disabled and Grayed Out" ("無効")
        # "Set Lock Mode to the Switch"
        n38 = property on="P1" class="Bool (strict)"("DisabledEnum"=w90) -> ()  [unwired: 2 in, 2 out]
        n39 = property on="P5" class="Bool (strict)"("DisabledEnum"=w90) -> ()  [unwired: 2 in, 2 out]
        n40 = property on="P7" class="Bool (strict)"("DisabledEnum"=w90) -> ()  [unwired: 2 in, 2 out]
        n41 = property on="P2" class="Bool (strict)"("DisabledEnum"=w90) -> ()  [unwired: 2 in, 2 out]
        n42 = property on="P6" class="Bool (strict)"("DisabledEnum"=w90) -> ()  [unwired: 2 in, 2 out]
        n43 = property on="P8" class="Bool (strict)"("DisabledEnum"=w90) -> ()  [unwired: 2 in, 2 out]
        n44 = property on="P3" class="Bool (strict)"("DisabledEnum"=w90) -> ()  [unwired: 2 in, 2 out]
        n45 = property on="EXIT" class="Bool (strict)"("DisabledEnum"=w90) -> ()  [unwired: 2 in, 2 out]
        n46 = property on="Export" class="Bool (strict)"("DisabledEnum"=w90) -> ()  [unwired: 2 in, 2 out]
        n47 = property on="P4" class="Bool (strict)"("DisabledEnum"=w90) -> ()  [unwired: 2 in, 2 out]
        n48 = case shown="True" w92 {
          tunnel: w90 -> [_ w101]
          frame False {
          }
          frame True {
            n49 = property on="Start" class="Bool (strict)"("DisabledEnum"=w101) -> ()  [unwired: 2 in, 2 out]
          }
        }
      }
      frame "SetPower" {
        # "Set power of the PMT-Module"
        n50 = local read "P1"() -> (w114:bool)
        n51 = Boolean To (0,1)(Boolean=w114) -> (0, 1=w113:i16)
        n52 = To Long Integer(number=w113) -> (32bit integer=w112:i32)
        n53 = call "Set HV.vi"("HV"=w112, "handle"=w115) -> ()  [unwired: 8 in, 2 out]
      }
      frame "SetIT" {
        # "Set internal time ....."
        n54 = local read "IT"() -> (w131:i32)
        n55 = To Long Integer(number=w131) -> (32bit integer=w132:i32)
        n56 = call "Set IT.vi"("IT"=w132, "handle"=w133) -> ()  [unwired: 8 in, 2 out]
        n57 = local write "P3"(FALSE ("P3")) -> ()
      }
      frame "SetRN" {
        # "Set read number ....."
        n58 = local read "RN"() -> (w149:i32)
        n59 = To Long Integer(number=w149) -> (32bit integer=w150:i32)
        n60 = call "Set RN.vi"("RN"=w150, "handle"=w151) -> ()  [unwired: 8 in, 2 out]
        n61 = local write "P5"(FALSE ("P3")) -> ()
      }
      frame "SetStepProp" {
        # "add the repeat step values for input and read here"
        # "Set Step SIze properties....."
        n62 = stacked-sequence {
          frame #0 {
            n63 = local read "WT"() -> (w174:i32)
            n64 = local read "ES"() -> (w173:i32)
            n65 = local read "SS"() -> (w175:i32)
            n66 = local read "EP"() -> (w176:i32)
            n67 = local read "SP"() -> (w177:i32)
            n68 = local write "SSD"(w175) -> ()
            n69 = local write "WTD"(w174) -> ()
            n70 = local write "ESD"(w173) -> ()
            n71 = local write "SPD"(w177) -> ()
            n72 = local write "EPD"(w176) -> ()
            n73 = local read "RS"() -> (w172:i32)
            n74 = local write "RSD"(w172) -> ()
          }
          frame #1 {
            n75 = local read "SP"() -> (w179:i32)
            n76 = local read "EP"() -> (w180:i32)
            n77 = local read "SS"() -> (w184:i32)
            n78 = local read "ES"() -> (w182:i32)
            n79 = Subtract(x=w180, y=w179) -> (x-y=w178:i32)
            n80 = Divide(x=w178, y=w184) -> (x/y=w183:dbl)
            n81 = Add(x=w183, y=w182) -> (x+y=w181:dbl)
            n82 = local write "SND"(w181) -> ()
          }
        }
        n83 = local write "P7"(FALSE) -> ()
      }
      frame "ReadPower" {
        # "Read power flag of the PMT-Module"
        n84 = local read "PowerD"() -> (w198:i32)
        n85 = call "Read HV.vi"("HV"=w198, "handle"=w197) -> ("HV out"=w196:i32)  [unwired: 7 in, 2 out]
        n86 = local write "PowerD"(w196) -> ()
        n87 = local write "P2"(FALSE ("P2")) -> ()
      }
      frame "ReadIT" {
        # "Read internal time of the PMT-Module"
        n88 = local read "ITD"() -> (w216:i32)
        n89 = call "Read IT.vi"("IT"=w216, "handle"=w215) -> ("IT out"=w214:i32)  [unwired: 7 in, 2 out]
        n90 = local write "ITD"(w214) -> ()
        n91 = local write "P4"(FALSE ("P4")) -> ()
      }
      frame "ReadRN" {
        # "Read data read number of the PMT-Module"
        n92 = local read "RND"() -> (w234:i32)
        n93 = call "Read RN.vi"("RN"=w234, "handle"=w233) -> ("RN out"=w231:i32)  [unwired: 7 in, 2 out]
        n94 = local write "RND"(w231) -> ()
        n95 = local write "P6"(FALSE ("P4")) -> ()
      }
      frame "ReadSN" {
        # "Read data sweep number of the Motorized stage"
        n96 = Increment(x=w241) -> (x+1=w242:i32)
        n97 = local write "SN"(w242) -> ()
      }
      frame "ReadSIN" {
        w256 = 0
        w258 = 0
        # "Clear Data DIM !"
        # "Read data sweep number of the Motorized stage"
        n98 = Initialize Array(w258, w258) -> (w257:i32[])
        n99 = local write "SN"(w256) -> ()
        n100 = Increment(x=w254) -> (x+1=w255:i32)
        n101 = local write "SIN"(w255) -> ()
      }
      frame "CountStart" {
        # "Conter Start!"
        n102 = local read "Correction"() -> (w281:bool)
        n103 = Boolean To (0,1)(Boolean=w281) -> (0, 1=w283:i16)
        n104 = To Long Integer(number=w283) -> (32bit integer=w282:i32)
        n105 = call "Count Start.vi"("Correction"=w282, "handle"=w284) -> ()  [unwired: 8 in, 2 out]
      }
      frame "CountStop" {
        w292 = FALSE ("Start")
        # "Add Auto Sweep button local variable here"
        # "Conter Stop!"
        n106 = local write "Auto-Sweep"(w292) -> ()
        n107 = local write "Stop"(w292) -> ()
        n108 = local write "Start"(w292) -> ()
        n109 = call "Count Stop.vi"("handle"=w303) -> ()  [unwired: 9 in, 2 out]
        n110 = Build Array (concatenate)(w301, "ActiveSwitch") -> (w300:string[])
      }
      frame "ReadData" {
        # "Read Data...."
        n111 = stacked-sequence {
          seq-local: [_ w332 _] -> [_ _ w342]
          seq-local: [_ w331 _] -> [_ _ w343]
          tunnel: w320 -> [_ w337 _]
          tunnel: w319 -> [_ _ w345]
          tunnel: [_ _ w344] -> w318
          tunnel: [_ w327 _] -> w317
          tunnel: w316 -> [_ w330 _]
          frame #0 {
            # "DB Clear!"
            n112 = Initialize Array(u32 0, 16 ("次元サイズ")) -> (w324:u32[])
            n113 = local write "DB"(w324) -> ()
          }
          frame #1 {
            n114 = local read "OLD"() -> (w334:i32)
            n115 = local read "GN"() -> (w336:i32)
            n116 = local read "DB"() -> (w335:u32[])
            n117 = call "Read Data.vi"("OLD"=w334, "DataBuf"=w335, "GateNum"=w336, "handle"=w337) -> ("OLD out"=w333:i32, "DataBuf out"=w331:u32[], "GateNum out"=w329:i32, "function return"=w332:u32)  [unwired: 3 in, 1 out]
            n118 = local write "OLD"(w333) -> ()
            n119 = local write "GN"(w329) -> ()
            n120 = local write "DB"(w331) -> ()
            n121 = Build Array(w329) -> (w328:i32[])
            n122 = Build Array (concatenate)(w330, w328) -> (w327:i32[])
          }
          frame #2 {
            # "Check Over Rang !"
            # "ADD Data DIM"
            # "Pickup Tans Data!"
            n123 = To Long Integer(number=w342) -> (32bit integer=w340:i32)
            n124 = local read "OLD"() -> (w339:i32)
            n125 = Array Subset(array=w343, length=w340) -> (w341:u32[])  [unwired: 1 in]
            n126 = Not Equal To 0?(x=w339) -> (x != 0?=w338:bool)
            n127 = local write "OVL"(w338) -> ()
            n128 = Build Array (concatenate)(w345, w341) -> (w344:u32[])
            n129 = local write "Graph"(w344) -> ()
          }
        }
      }
      frame "AutoReadData" {
        # "Read Data...."
        n130 = stacked-sequence {
          tunnel: w351 -> [w373 _]
          tunnel: [w370 _] -> w350
          tunnel: w349 -> [w372 _]
          tunnel: w348 -> [w371 w375]
          frame #0 {
            n131 = Build Array (concatenate)(w372, w373) -> (w370:i32[])
            n132 = Bundle By Name("Y"=w371) -> (w368:waveform(i32))  [unwired: 1 in]
            n133 = Bundle By Name("Y"=w370) -> (w364:waveform(i32))  [unwired: 1 in]
            n134 = Get Waveform Attribute(6:"Sweep Meaned", 7:w368) -> (3:w367:waveform(i32))  [unwired: 2 in, 3 out]
            n135 = Get Waveform Attribute(6:"Mean Data", 7:w364) -> (3:w365:waveform(i32))  [unwired: 2 in, 3 out]
            n136 = Bundle(w367, w365) -> (w363:cluster{waveform(i32), waveform(i32)})  [unwired: 1 in]
            n137 = local write "Sweep Graph"(w370) -> ()
            n138 = Cluster To Array(cluster=w363) -> (array=w362:waveform(i32)[])
            n139 = local write "Multiplot"(w362) -> ()
          }
          frame #1 {
            n140 = local read "SIN"() -> (w376:i32)
            n141 = Equal To 0?(x=w376) -> (x = 0?=w377:bool)
            n142 = case shown="False" w377 {
              tunnel: w375 -> [w378 _]
              tunnel: [w378 w379] -> w374
              frame False {
              }
              frame True {
                n143 = local read "Sweep Graph"() -> (w379:u32[])
              }
            }
            n144 = local write "Cycled Mean Graph"(w374) -> ()
          }
        }
      }
      frame "CountInit" {
        w391 = 0
        # "Auto"
        # "Clear Data DIM !"
        n145 = Initialize Array(w391, w391) -> (w389:i32[])
        n146 = Build Array("LockSwitch", "ReadRN", "CountStart", "ReadData", "CheckNumber") -> (w392:string[])
        n147 = Build Array (concatenate)(w398, w392) -> (w397:string[])
      }
      frame "AutoCount|nit!" {
        w418 = 0
        # "Edit caser for SIN and SIND"
        # "Clear Data DIM !"
        n148 = Initialize Array(w418, w418) -> (w417:i32[])
        n149 = local read "SND"() -> (w405:i32)
        n150 = local read "SN"() -> (w410:i32)
        n151 = Increment(x=w405) -> (x+1=w406:i32)
        n152 = Less?(x=w410, y=w406) -> (x < y?=w409:bool)
        n153 = case shown="True" w409 {
          tunnel: w408 -> [w425 w428]
          tunnel: [w423 w427] -> w407
          frame False {
            n154 = Build Array("AutoReadData", "AutoCheckNumber") -> (w424:string[])
            n155 = Build Array (concatenate)(w425, w424) -> (w423:string[])
          }
          frame True {
            n156 = Build Array("LockSwitch", "ReadRN", "CountStart", "ReadData", "AutoCheckNumber") -> (w434:string[])
            n157 = Build Array (concatenate)(w428, w434) -> (w427:string[])
          }
        }
      }
      frame "CheckNumber" {
        # "Add append"
        # "Add Case Strucutre outside\nsimilar to GN,"
        # "Check RN and Data lenbgth,Stop Switch ......"
        n158 = local read "Stop"() -> (w446:bool)
        n159 = local read "GN"() -> (w447:i32)
        n160 = Decrement(x=w449) -> (x-1=w448:i32)
        n161 = Less?(x=w447, y=w448) -> (x < y?=w453:bool)
        n162 = case shown="True" w453 {
          tunnel: [w459 w461] -> w450
          tunnel: w446 -> [_ w460]
          frame False {
            # "\"MotorJog\"; here"
            # "Move \"Active Swith\" to False Condition of Position Number"
            # "Add \"AutoExport Run\" here"
            n163 = local write "Start"(FALSE ("Start")) -> ()
            n164 = Build Array("CountStop", "ActiveSwitch") -> (w459:string[])
          }
          frame True {
            n165 = case shown="False" w460 {
              tunnel: [w463 w465] -> w461
              frame False {
                n166 = Build Array("ReadData", "CheckNumber") -> (w463:string[])
              }
              frame True {
                n167 = Build Array("CountStop") -> (w465:string[])
              }
            }
          }
        }
        n168 = Build Array (concatenate)(w451, w450) -> (w452:string[])
      }
      frame "AutoCheckNumber" {
        # "Add another Case structure to add the repeat cycle SIN and SIND over the SN and SND"
        # "Add Case Strucutre outside\nsimilar to GN,"
        n169 = local read "SIND"() -> (w469:i32)
        n170 = local read "Stop"() -> (w481:bool)
        n171 = local read "SIN"() -> (w470:i32)
        n172 = Less?(x=w470, y=w469) -> (x < y?=w468:bool)
        n173 = case shown="True" w468 {
          tunnel: [w489 w499] -> w483
          tunnel: w482 -> [_ w498]
          tunnel: w481 -> [_ w497]
          tunnel: [TRUE w496] -> w476
          frame False {
            (unwired) "AutoExportMeanSweep"
            (unwired) "AutoExportSweep"
            w491 = FALSE
            # "Removed to check the difference"
            n174 = local write "Auto-Sweep"(w491) -> ()
            n175 = local write "Start"(w491) -> ()
            n176 = Build Array("CountStop", "ActiveSwitch") -> (w489:string[])
          }
          frame True {
            # "Add append"
            # "Check RN and Data lenbgth,Stop Switch ......"
            n177 = local read "SND"() -> (w493:i32)
            n178 = local read "SN"() -> (w495:i32)
            n179 = Less?(x=w495, y=w493) -> (x < y?=w494:bool)
            n180 = case shown="False" w494 {
              tunnel: [w505 w513] -> w499
              tunnel: w498 -> [_ w512]
              tunnel: w497 -> [_ w509]
              tunnel: [FALSE w508] -> w496
              frame False {
                # "ActiveSwitch"
                # "AutoCheckSweepIter"
                n181 = Build Array("CountStop", "AutoExportSweep", "AutoExportMeanSweep", "ReadSIN", "SetPosition", "AutoCount|nit!") -> (w505:string[])
              }
              frame True {
                n182 = local read "GN"() -> (w510:i32)
                n183 = Decrement(x=w512) -> (x-1=w511:i32)
                n184 = Less?(x=w510, y=w511) -> (x < y?=w514:bool)
                n185 = case shown="False" w514 {
                  tunnel: [w516 w532] -> w513
                  tunnel: w509 -> [w517 w531]
                  tunnel: [w515 w530] -> w508
                  frame False {
                    # "\"MotorJog\"; here"
                    # "Move \"Active Swith\" to False Condition of Position Number"
                    # "Add \"AutoExport Run\" here"
                    n186 = case shown="False" w517 {
                      tunnel: [w523 w528] -> w516
                      tunnel: [FALSE TRUE] -> w515
                      frame False {
                        n187 = Build Array("CountStop", "AutoExportRun", "AutoReadData", "ReadSN", "MotorJog", "AutoCount|nit!") -> (w523:string[])
                      }
                      frame True {
                        n188 = local write "Auto-Sweep"(TRUE) -> ()
                        n189 = Build Array("CountStop") -> (w528:string[])
                      }
                    }
                  }
                  frame True {
                    n190 = case shown="False" w531 {
                      tunnel: [w535 w539] -> w532
                      tunnel: [FALSE TRUE] -> w530
                      frame False {
                        n191 = Build Array("ReadData", "AutoCheckNumber") -> (w535:string[])
                      }
                      frame True {
                        n192 = Build Array("CountStop") -> (w539:string[])
                        n193 = local write "Auto-Sweep"(TRUE) -> ()
                      }
                    }
                  }
                }
              }
            }
          }
        }
        n194 = Build Array (concatenate)(w484, w483) -> (w485:string[])
      }
      frame "Export" {
        # "For Auto Export also add mean waveform"
        # "Get mean Data into 1D array Shift register for waveform"
        # "Gate Number is just number of count measurements"
        # "time...using array size"
        # "time...using array size"
        n195 = Array Size(array=w558) -> (size(s)=w570:i32)
        n196 = for {
          N: w570 -> [_]
          tunnel: [w576] -> w557 mode=indexing
          i -> [w578]
          n197 = local read "ITD"() -> (w580:i32)
          n198 = Add(x=1, y=w578) -> (x+y=w579:i32)
          n199 = Multiply(x=w580, y=w579) -> (x*y=w576:i32)
        }
        n200 = call <vilib>:"Std Deviation and Variance.vi"("X"=w558) -> ("mean"=w551:dbl, "standard deviation"=w550:dbl)  [unwired: 1 in, 1 out]
        n201 = Build Array(w551, w550) -> (w549:dbl[])
        n202 = Build Array(w553, w557, w558) -> (w568:u32[][])
        n203 = call-poly <vilib>:"Write Delimited Spreadsheet.vi"("1D data"=string[] ["Gate  No.", "Time [ms]", "Counts"], "append to file? (new file:F)"=FALSE, "transpose? (no:F)"=FALSE) -> ("new file path (Not A Path if cancelled)"=w567:path)  [unwired: 11 in, 1 out]
        n204 = call-poly <vilib>:"Write Delimited Spreadsheet.vi"("file path (dialog if empty)"=w567, "2D data"=w568, "append to file? (new file:F)"=TRUE, "transpose? (no:F)"=TRUE) -> ("new file path (Not A Path if cancelled)"=w563:path)  [unwired: 10 in, 1 out]
        n205 = call-poly <vilib>:"Write Delimited Spreadsheet.vi"("file path (dialog if empty)"=w563, "1D data"=string[] ["Mean", "Std. Dev."], "append to file? (new file:F)"=TRUE, "transpose? (no:F)"=FALSE) -> ("new file path (Not A Path if cancelled)"=w559:path)  [unwired: 10 in, 1 out]
        n206 = call-poly <vilib>:"Write Delimited Spreadsheet.vi"("file path (dialog if empty)"=w559, "1D data"=w549, "append to file? (new file:F)"=TRUE, "transpose? (no:F)"=FALSE) -> ()  [unwired: 10 in, 2 out]
        n207 = local write "Export"(FALSE) -> ()
      }
      frame "AutoExportRun" {
        # "For Auto Export also add mean waveform"
        # "Get mean Data into 1D array Shift register for waveform"
        # "Gate Number is just number of count measurements"
        # "time...using array size"
        # "time...using array size"
        n208 = Array Size(array=w606) -> (size(s)=w618:i32)
        n209 = for {
          N: w618 -> [_]
          tunnel: [w629] -> w605 mode=indexing
          i -> [w631]
          n210 = local read "ITD"() -> (w633:i32)
          n211 = Add(x=1, y=w631) -> (x+y=w632:i32)
          n212 = Multiply(x=w633, y=w632) -> (x*y=w629:i32)
        }
        n213 = flat-sequence {
          tunnel: w591 -> [w628]
          tunnel: [w624] -> w590
          frame #0 {
            n214 = local read "SS"() -> (w627:i32)
            n215 = Multiply(x=w628, y=w627) -> (x*y=w625:i32)
            n216 = local read "SP"() -> (w626:i32)
            n217 = Add(x=w626, y=w625) -> (x+y=w624:i32)
          }
        }
        n218 = call <vilib>:"Std Deviation and Variance.vi"("X"=w606) -> ("mean"=w582:dbl, "standard deviation"=w599:dbl)  [unwired: 1 in, 1 out]
        n219 = To Long Integer(number=w582) -> (32bit integer=w581:i32)
        n220 = Build Array(w582, w599) -> (w598:dbl[])
        n221 = Number To Decimal String(number=w590) -> (decimal integer string=w589:string)  [unwired: 1 in]
        n222 = Build Array(w601, w605, w606) -> (w616:u32[][])
        n223 = Build Array (concatenate)(string[] ["Angle (deg)"], w589) -> (w587:string[])
        n224 = call-poly <vilib>:"Write Delimited Spreadsheet.vi"("file path (dialog if empty)"=w595, "1D data"=w587, "append to file? (new file:F)"=TRUE, "transpose? (no:F)"=FALSE) -> ("new file path (Not A Path if cancelled)"=w594:path)  [unwired: 10 in, 1 out]
        n225 = call-poly <vilib>:"Write Delimited Spreadsheet.vi"("file path (dialog if empty)"=w594, "1D data"=string[] ["Gate  No.", "Time [ms]", "Counts"], "append to file? (new file:F)"=TRUE, "transpose? (no:F)"=FALSE) -> ("new file path (Not A Path if cancelled)"=w615:path)  [unwired: 10 in, 1 out]
        n226 = call-poly <vilib>:"Write Delimited Spreadsheet.vi"("file path (dialog if empty)"=w615, "2D data"=w616, "append to file? (new file:F)"=TRUE, "transpose? (no:F)"=TRUE) -> ("new file path (Not A Path if cancelled)"=w611:path)  [unwired: 10 in, 1 out]
        n227 = call-poly <vilib>:"Write Delimited Spreadsheet.vi"("file path (dialog if empty)"=w611, "1D data"=string[] ["Mean", "Std. Dev."], "append to file? (new file:F)"=TRUE, "transpose? (no:F)"=FALSE) -> ("new file path (Not A Path if cancelled)"=w607:path)  [unwired: 10 in, 1 out]
        n228 = call-poly <vilib>:"Write Delimited Spreadsheet.vi"("file path (dialog if empty)"=w607, "1D data"=w598, "append to file? (new file:F)"=TRUE, "transpose? (no:F)"=FALSE) -> ("new file path (Not A Path if cancelled)"=w597:path)  [unwired: 10 in, 1 out]
        n229 = local write "Export"(FALSE) -> ()
      }
      frame "AutoExportSweep" {
        # "For Auto Export also add mean waveform"
        # "Get mean Data into 1D array Shift register for waveform"
        # "Gate Number is just number of count measurements"
        # "time...using array size"
        # "time...using array size"
        n230 = Array Size(array=w636) -> (size(s)=w665:i32)
        n231 = for {
          N: w665 -> [_]
          tunnel: [w683] -> w652 mode=indexing
          i -> [w680]
          n232 = local read "SS"() -> (w684:i32)
          n233 = Multiply(x=w684, y=w680) -> (x*y=w681:i32)
          n234 = local read "SP"() -> (w682:i32)
          n235 = Add(x=w682, y=w681) -> (x+y=w683:i32)
        }
        n236 = call <vilib>:"Std Deviation and Variance.vi"("X"=w636) -> ("mean"=w634:dbl, "standard deviation"=w646:dbl)  [unwired: 1 in, 1 out]
        n237 = To Long Integer(number=w634) -> (32bit integer=w635:i32)
        n238 = Build Array(w634, w646) -> (w645:dbl[])
        n239 = Array Size(array=w636) -> (size(s)=w640:i32)
        n240 = Build Array(w652, w636) -> (w663:i32[][])
        n241 = for {
          N: w640 -> [_]
          tunnel: [w673] -> w639 mode=indexing
          tunnel: [w671] -> w638 mode=indexing
          tunnel: w636 -> [w675] mode=indexing
          i -> [w676]
          n242 = local read "Cycled Mean Graph"() -> (w677:u32[])
          n243 = Index Array(array=w677, index=w676) -> (element=w679:u32)
          n244 = Build Array(w679, w675) -> (w678:u32[])
          n245 = call <vilib>:"Std Deviation and Variance.vi"("X"=w678) -> ("mean"=w674:dbl, "standard deviation"=w672:dbl)  [unwired: 1 in, 1 out]
          n246 = To Long Integer(number=w672) -> (32bit integer=w671:i32)
          n247 = To Long Integer(number=w674) -> (32bit integer=w673:i32)
        }
        n248 = call-poly <vilib>:"Write Delimited Spreadsheet.vi"("file path (dialog if empty)"=w642, "1D data"=string[] ["Angle Itr.", "Counts Mean", ""], "append to file? (new file:F)"=TRUE, "transpose? (no:F)"=FALSE) -> ("new file path (Not A Path if cancelled)"=w662:path)  [unwired: 10 in, 1 out]
        n249 = call-poly <vilib>:"Write Delimited Spreadsheet.vi"("file path (dialog if empty)"=w662, "2D data"=w663, "append to file? (new file:F)"=TRUE, "transpose? (no:F)"=TRUE) -> ("new file path (Not A Path if cancelled)"=w658:path)  [unwired: 10 in, 1 out]
        n250 = call-poly <vilib>:"Write Delimited Spreadsheet.vi"("file path (dialog if empty)"=w658, "1D data"=string[] ["Mean", "Std. Dev."], "append to file? (new file:F)"=TRUE, "transpose? (no:F)"=FALSE) -> ("new file path (Not A Path if cancelled)"=w654:path)  [unwired: 10 in, 1 out]
        n251 = call-poly <vilib>:"Write Delimited Spreadsheet.vi"("file path (dialog if empty)"=w654, "1D data"=w645, "append to file? (new file:F)"=TRUE, "transpose? (no:F)"=FALSE) -> ("new file path (Not A Path if cancelled)"=w644:path)  [unwired: 10 in, 1 out]
        n252 = local write "Export"(FALSE) -> ()
      }
      frame "AutoExportMeanSweep" {
        # "For Auto Export also add mean waveform"
        # "Get mean Data into 1D array Shift register for waveform"
        # "Gate Number is just number of count measurements"
        # "time...using array size"
        n253 = Array Size(array=w691) -> (size(s)=w709:i32)
        n254 = for {
          N: w709 -> [_]
          tunnel: [w718] -> w702 mode=indexing
          i -> [w715]
          n255 = local read "SS"() -> (w719:i32)
          n256 = Multiply(x=w719, y=w715) -> (x*y=w716:i32)
          n257 = local read "SP"() -> (w717:i32)
          n258 = Add(x=w717, y=w716) -> (x+y=w718:i32)
        }
        n259 = Build Array(w702, w691, w692) -> (w707:i32[][])
        n260 = local write "Export"(FALSE) -> ()
        n261 = call-poly <vilib>:"Write Delimited Spreadsheet.vi"("file path (dialog if empty)"=w687, "1D data"=string[] ["Mean of Sweep", "", ""], "append to file? (new file:F)"=TRUE, "transpose? (no:F)"=FALSE) -> ("new file path (Not A Path if cancelled)"=w686:path)  [unwired: 10 in, 1 out]
        n262 = call-poly <vilib>:"Write Delimited Spreadsheet.vi"("file path (dialog if empty)"=w686, "1D data"=string[] ["Angle Itr.", "Counts Mean", "Std. Dev."], "append to file? (new file:F)"=TRUE, "transpose? (no:F)"=FALSE) -> ("new file path (Not A Path if cancelled)"=w706:path)  [unwired: 10 in, 1 out]
        n263 = call-poly <vilib>:"Write Delimited Spreadsheet.vi"("file path (dialog if empty)"=w706, "2D data"=w707, "append to file? (new file:F)"=TRUE, "transpose? (no:F)"=TRUE) -> ("new file path (Not A Path if cancelled)"=w693:path)  [unwired: 10 in, 1 out]
      }
      frame "AutoSweep" {
        # "Remove the sequence stack"
        # "Remove and move RSD and sind to different case"
        # "1. Create a file path (Send two strings, \"SetPosition\" and \"AutoCount|nit!\")\n2. Send to \"SetPosition\"\n2.1. Will create a Position Number Shift register\n2.2. Move stage to initial position, allow time to complete movement or add delay\n3. Send to \"AutoCount|nit!\"\n3.1. \"AutoCount|nit!\" is clone of \"Count|nit!\" but sends to \"AutoCheckNumber\", not \"CheckNumber\n3.1.1. \"AutoCheckNumber\" will check if end position, or run condition is met then send \"CountStop\" and \"ActiveSwitch\"\n3.1.2. \"AutoCheck Number\" will allow \"CountStop\" to be sent via Stop Boolean\n3.1.3. \"AutoCheckNumber\" will upon END of one run will run \"AutoExportRun\" to set file path\n3.1.3.1. \"AutoExportRun\" will add a data point to Mean Waveform after Count Stop\n3.1.4. \"AutoCheckNumber\" will upon END of sweep will run \"AutoExportSweep\" then issue \"ActiveSwitch\"\n3.1.4.1. \"AutoExportSweep\" will append final Mean Sweep waveform to file path before \"CountStop\";\"ActiveSwitch\"\n4. If End condition not met; \"MotorJog\"; \"AutoCount|nit!\"....repeats\n4.1. Will move to next position by set increment, with .net code, add delay to allow it to arrive at position"
        # "Create a File path here\nSend switch case string \"SetPosition\", which has a position number switch register"
        # "1.Position Set, create a file path\n2. Count|nit!---duplicate and create auto counter, add read sweep data for auto read\n2.0.1Checknumber end, change active switch to Auto export\n3. Auto Export ... need to make \n3.0.2Auto Export end, send to read sweep data (mean, stdev for per sweep)\n3.Export\n4.check end position, check end condition met\n5.met>end;not end >continue\n6. Jog motor\n7.repeat from 2."
        # "Create Motor Controls for setting Homing, Step size for angle, idle time(if required),"
        n264 = stacked-sequence {
          seq-local: [w735 _ _ _] -> [_ _ w739 _]
          tunnel: [_ _ w739 _] -> w720
          tunnel: [_ _ w737 _] -> w723
          tunnel: w722 -> [_ _ _ w741]
          tunnel: [_ _ _ w740] -> w721
          frame #0 {
            w735 = 0
            n265 = local write "SIN"(w735) -> ()
            n266 = local write "SN"(w735) -> ()
          }
          frame #1 {
            n267 = local read "RSD"() -> (w736:i32)
            n268 = local write "SIND"(w736) -> ()
          }
          frame #2 {
            n269 = call-poly <vilib>:"Write Delimited Spreadsheet.vi"("append to file? (new file:F)"=FALSE) -> ("new file path (Not A Path if cancelled)"=w737:path)  [unwired: 13 in, 1 out]
          }
          frame #3 {
            n270 = Build Array("SetPosition", "AutoCount|nit!") -> (w744:string[])
            n271 = Build Array (concatenate)(w741, w744) -> (w740:string[])
          }
        }
      }
      frame "MotorJog" {
        # "Move position by set increment"
        # "Add a test Jog?"
        # "Put thor labs net code here"
        n272 = stacked-sequence {
          tunnel: w753 -> [w766 w771]
          frame #0 {
            n273 = local read "SSD"() -> (w765:i32)
            n274 = invoke class="KCubeDCServo" method="MoveRelative"(reference=w766, "direction"=1, "stepSize"=w765, "waitTimeout"=0) -> ()  [unwired: 2 in, 6 out]
            n275 = local read "WT"() -> (w763:i32)
            n276 = Wait (ms)(milliseconds to wait=w763) -> ()  [unwired: 1 out]
          }
          frame #1 {
            n277 = invoke class="KCubeDCServo" method="GetPositionCounter"(reference=w771) -> ("GetPositionCounter"=w769:i32)  [unwired: 2 in, 2 out]
            n278 = Divide(x=w769, y=1919.6418578623338) -> (x/y=w767:dbl)
            n279 = Wait (ms)(milliseconds to wait=50) -> ()  [unwired: 1 out]
            n280 = local write "PC"(w767) -> ()
          }
        }
        n281 = local write "P8"(FALSE) -> ()
      }
      frame "SetPosition" {
        # "Add a waveform property node to clear history of the graph for user friendliness"
        n282 = stacked-sequence {
          tunnel: w779 -> [w789 w794 w799]
          frame #0 {
            n283 = local read "SPD"() -> (w788:i32)
            n284 = invoke class="KCubeDCServo" method="SetMoveAbsolutePosition"(reference=w789, "position"=w788) -> ()  [unwired: 2 in, 4 out]
          }
          frame #1 {
            n285 = invoke class="KCubeDCServo" method="MoveAbsolute"(reference=w794, "waitTimeout"=25000) -> ()  [unwired: 2 in, 4 out]
            n286 = local read "WT"() -> (w790:i32)
            n287 = Add(x=w790, y=20000) -> (x+y=w791:i32)
            n288 = Wait (ms)(milliseconds to wait=w791) -> ()  [unwired: 1 out]
          }
          frame #2 {
            n289 = invoke class="KCubeDCServo" method="GetPositionCounter"(reference=w799) -> ("GetPositionCounter"=w796:i32)  [unwired: 2 in, 2 out]
            n290 = Divide(x=w796, y=1919.6418578623338) -> (x/y=w795:dbl)
            n291 = local write "PC"(w795) -> ()
            n292 = Wait (ms)(milliseconds to wait=50) -> ()  [unwired: 1 out]
          }
        }
      }
      frame "", "Idle" {
        n293 = event shown="[7] \"P6\": Value Change" {
          selector: _ -> [_ _ _ _ _ _ _ _ _ _ _ _ _]
          dyn-events: _ -> [_ _ _ _ _ _ _ _ _ _ _ _ _]
          timeout: _ -> [_ _ _ _ _ _ _ _ _ _ _ _ _]
          tunnel: w814 -> [w820 w823 w826 w830 w834 w838 w842 w846 w849 w851 w854 w857 w860]
          tunnel: [w818 w822 w825 w829 w833 w837 w841 w845 w848 w850 w853 w856 w861] -> w812
          event Menu Selection (User) {
            n294 = event-data() -> ("ItemTag"=w819:string)  [unwired: 1 out]
            n295 = Build Array (concatenate)(w820, w819) -> (w818:string[])
          }
          event "EXIT": Value Change {
            n296 = event-data() -> ()  [unwired: 7 out]
            n297 = Build Array (concatenate)(w823, "Exit") -> (w822:string[])
          }
          event "P1": Value Change {
            n298 = event-data() -> ()  [unwired: 7 out]
            n299 = Build Array (concatenate)(w826, "SetPower") -> (w825:string[])
          }
          event "P2": Value Change {
            n300 = event-data() -> ()  [unwired: 7 out]
            n301 = Build Array (concatenate)(w830, "ReadPower") -> (w829:string[])
            n302 = Wait (ms)(milliseconds to wait=u32 200 ("ミリ秒待機時間")) -> ()  [unwired: 1 out]
          }
          event "P3": Value Change {
            n303 = event-data() -> ()  [unwired: 7 out]
            n304 = Build Array (concatenate)(w834, "SetIT") -> (w833:string[])
            n305 = Wait (ms)(milliseconds to wait=u32 200 ("ミリ秒待機時間")) -> ()  [unwired: 1 out]
          }
          event "P4": Value Change {
            n306 = event-data() -> ()  [unwired: 7 out]
            n307 = Build Array (concatenate)(w838, "ReadIT") -> (w837:string[])
            n308 = Wait (ms)(milliseconds to wait=u32 200 ("ミリ秒待機時間")) -> ()  [unwired: 1 out]
          }
          event "P5": Value Change {
            n309 = event-data() -> ()  [unwired: 7 out]
            n310 = Build Array (concatenate)(w842, "SetRN") -> (w841:string[])
            n311 = Wait (ms)(milliseconds to wait=u32 200 ("ミリ秒待機時間")) -> ()  [unwired: 1 out]
          }
          event "P6": Value Change {
            n312 = event-data() -> ()  [unwired: 7 out]
            n313 = Build Array (concatenate)(w846, "ReadRN") -> (w845:string[])
            n314 = Wait (ms)(milliseconds to wait=u32 200 ("ミリ秒待機時間")) -> ()  [unwired: 1 out]
          }
          event "Start": Value Change {
            n315 = event-data() -> ()  [unwired: 7 out]
            n316 = Build Array (concatenate)(w849, "CountInit") -> (w848:string[])
          }
          event "Export": Value Change {
            n317 = event-data() -> ()  [unwired: 7 out]
            n318 = Build Array (concatenate)(w851, "Export") -> (w850:string[])
          }
          event "P7": Value Change {
            n319 = event-data() -> ()  [unwired: 7 out]
            n320 = Build Array (concatenate)(w854, "SetStepProp") -> (w853:string[])
          }
          event "P8": Value Change {
            n321 = event-data() -> ()  [unwired: 7 out]
            n322 = Build Array (concatenate)(w857, "MotorJog") -> (w856:string[])
          }
          event "Auto-Sweep": Value Change {
            n323 = event-data() -> ()  [unwired: 7 out]
            n324 = Build Array (concatenate)(w860, "AutoSweep") -> (w861:string[])
            n325 = Wait (ms)(milliseconds to wait=200) -> ()  [unwired: 1 out]
          }
        }
        n326 = Build Array (concatenate)("", w812) -> (w811:string[])
      }
      frame "Error", Default {
        n327 = Concatenate Strings("Error  Case Name .....", "\r\n", w873) -> (w875:string)
        n328 = One Button Dialog(message=w875) -> (true=w874:bool)  [unwired: 1 out]
        n329 = stacked-sequence {
          tunnel: w874 -> [_]
          frame #0 {
            n330 = Stop() -> ()  [unwired: 1 out]
          }
        }
      }
      frame "Exit" {
        # "See you again ......"
        n331 = call "Close.vi"("Handle"=w893) -> ()  [unwired: 9 in, 2 out]
      }
    }
    n332 = Divide(x=w19, y=1919.6418578623338) -> (x/y=w18:dbl)
    n333 = local write "PC"(w18) -> ()
    n334 = call "SM_CaseErase.vi"("Input"=w38) -> ("Output"=w37:string[])  [unwired: 10 out]
  }
  n335 = invoke class="KCubeDCServoControl" method="CloseDevice"(reference=w6) -> ()  [unwired: 2 in, 3 out]
